vi "GEA2 Extract 2015 Washer.vi"(6 "ERD Cross Reference List":T1[][](array[typedef]) {"ERD Number" format="%.0x"}, 7 "Enable Diagnostic Data":T3, 8 "Error In":errorcluster, 9 "ERD Number":u16 format="%x", 10 "Data":string, 11 "ERD Headers":string[](array[string])) -> (0 "Error Out":errorcluster, 3 "Array":string[][](array[string]))   [LabVIEW 2016, in "GEA2_Toolkit.lvlib"]
uses:
  library/GEA2_Toolkit.lvlib
  Washer HCC/Washer HCC NEWFI/Type Definitions/HCC Washer Types.ctl
  type defs/ERD Read Data In.ctl
  type defs/Data Type.ctl
panel:
  in  "Header Array (Debug)":string[](array[string])=["Critical Major (0x0100)", "Critical Minor (0x0100)", "Non-Critical Major (0x0100)", "Non-Critical Minor (0x0100)", "Daily Revision (0x0100)", "Cycle Count (0x008E)", "XML Critical Major (0xF014)", "XML Critical Minor (0xF014)", "XML Non-Critical Major (0xF014)", "XML Non-Critical Minor (0xF014)", "Available Free Stack % (0xF026)", "Extra Rinse (0xF032)", "Deep Rinse_Fabric Softener (0xF033)", "My Cycle (0xF034)", "Soil Level (0x2015)", "Spin Level (0xF035)", "Stain (0xF036)", "Temperature Level (0xF037)", "Load Size (0xF038)", "Machine State (0xF039)", "Cycle Selected (0xF03B)", "Delay Time (0x2010)", "Soak Time (0xF03C)", "Auto Soak Level (0xF04B)", "Deep Fill (0xF04F)", "Warm Rinse (0xF050)", "Remaining Cycle Time(s) (0xF061)", "Wet Load Gallons (0xF068)", "Tub Volume Gallons (0xF069)", "Pressure (inches of H20) (0xF06A)", "Target Gallons (0xF06D)", "Load Type (0xF06E)", "Lid Switch (0xF06F)", "Hot Water Valve (0xF09C)", "Cold Water Valve (0xF09C)", "Spray_Rinse Valve (0xF09C)", "Fabric Softener Valve (0xF09C)", "Lid Lock Req State (0xF072)", "Lid Lock Status (0xF073)", "Cycle Engine State (0xF074)", "Current Water Temperature (°F) (0xF077)", "Drain Pump (0xF09A)", "Recirculating Pump (0xF079)", "Sub-Cycle (0xF07B)", "Target Level Inches (0xF07D)", "Valve Relay (0xF09B)", "Lid Lock FB (0xF080)", "Target Bath Temperature (°F) (0xF082)", "Current Bath Temperature (°F) (0xF083)", "Cold Inlet Temperature (°F) (0xF084)", "Hot Inlet Temperature (°F) (0xF085)", "Warm Inlet Temperature (°F) (0xF086)", "Hot Gallons (0xF087)", "Cold Gallons (0xF087)", "Hot Seg Valve Time (0xF088)", "Cold Seg Valve Time (0xF088)", "Child Safety (0xF089)", "Segment Gallons (0xF08A)", "Ramp Average Current (0xF09E)", "Coast Line Voltage (0xF09F)", "Ramp Speed (0xF0A0)", "Ramp Time (0xF0A1)", "Coast Time (0xF0A2)", "Dry Load Size (0xF0A3)", "Folding in Acceleration (0xF0A4)", "Max Jerk In Acceleration (0xF0A5)", "Max Jerk In S-S (0xF0A6)", "Shaft Speed (RPM) (0xF0A8)", "Basket Speed (RPM) (0xF0A9)", "Current RMS (Amps) (0xF0AB)", "Target Speed (RPM) (0xF0AC)", "Motor Mode (0xF0B1)", "OOB Detected in Acceleration (0xF0B3)", "OOB Detected in S-S (0xF0B4)", "OOB ReDistribution Required (0xF0B5)", "Motor Profile Status (0xF0B7)", "Motor Profile (0xF0B7)", "Mode Shift Status (0xFF22)", "ME Relay (0xF0BE)", "Mode Shift FB (0xF0BF)", "MS Motor (0xF0C0)", "Partial Coast Time (0xF0C6)", "Ramp Line Voltage (0xF0C7)", "Personality (0xFF00)", "Reset Source (0xFF02)", "DC Bus Voltage RMS value (0xF0C4)"]
  out "ERD Number 2":u16 format="%x"
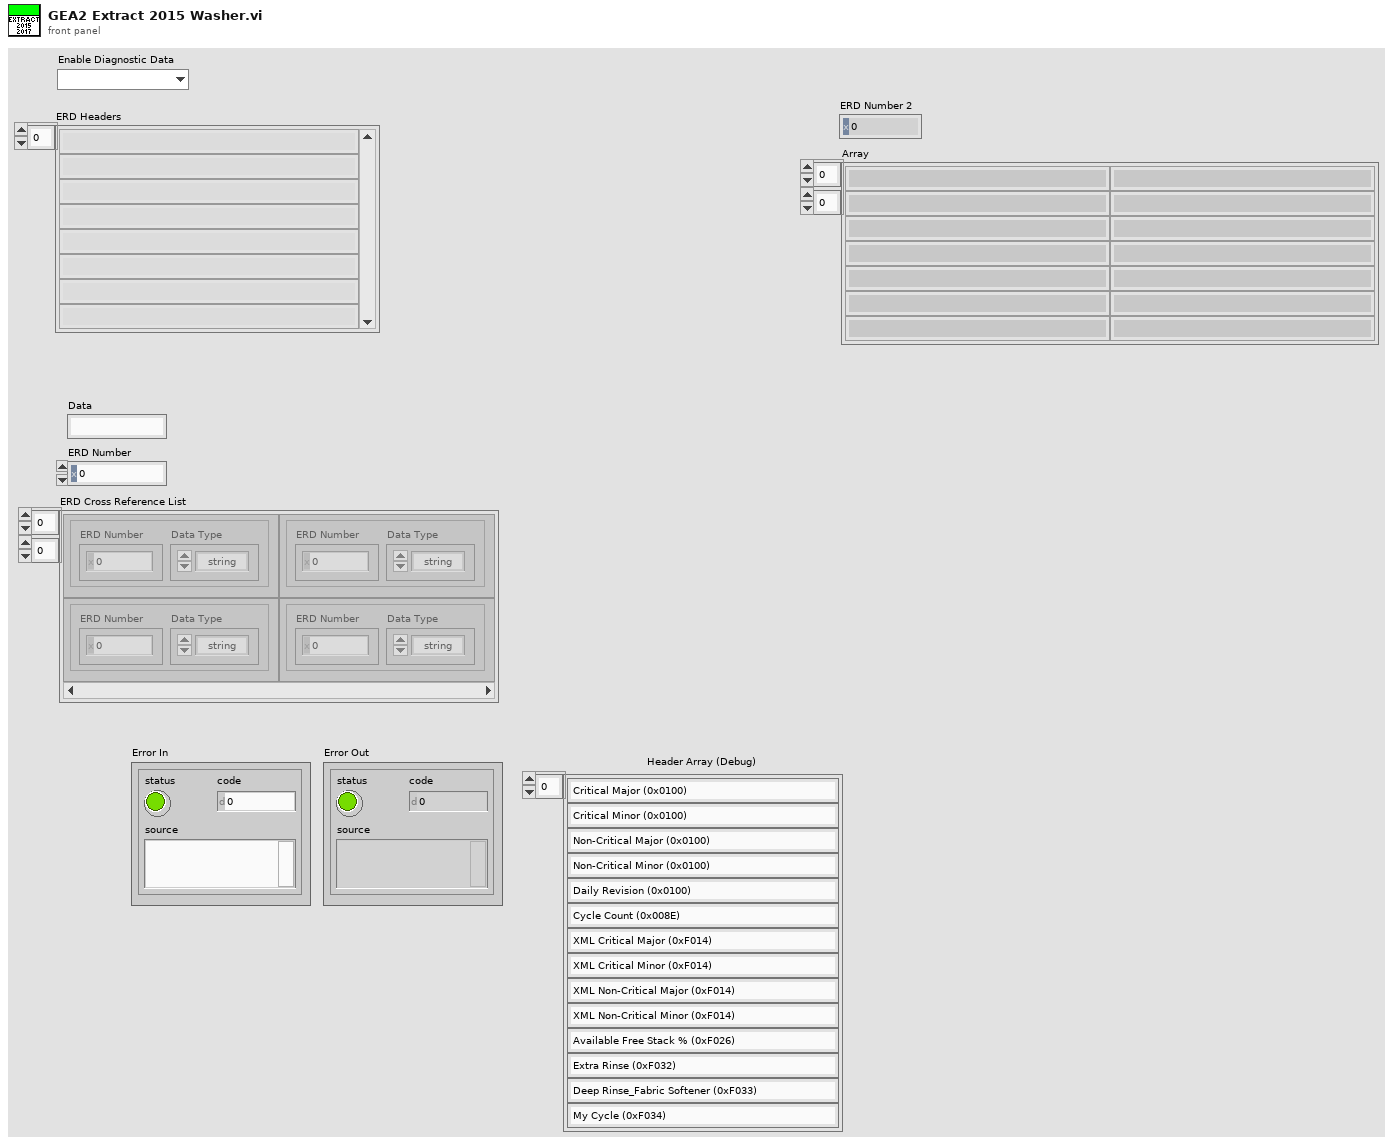
[diagram p1: front panel]
types:
  T1 = typedef "GEA2_Toolkit.lvlib/ERD Read Data In.ctl" = cluster{"ERD Number":u16, "Data Type":T2}
  T2 = typedef "GEA2_Toolkit.lvlib/Data Type.ctl" = enum16{"string", "boolean", "uint8_t", "uint16_t", "uint32_t", "uint64_t"}
  T3 = typedef "HCC Washer Types.ctl" = enum16{"", "Viper Washer", "Hawk Washer", "2015 Washer", "2017 Washer"}
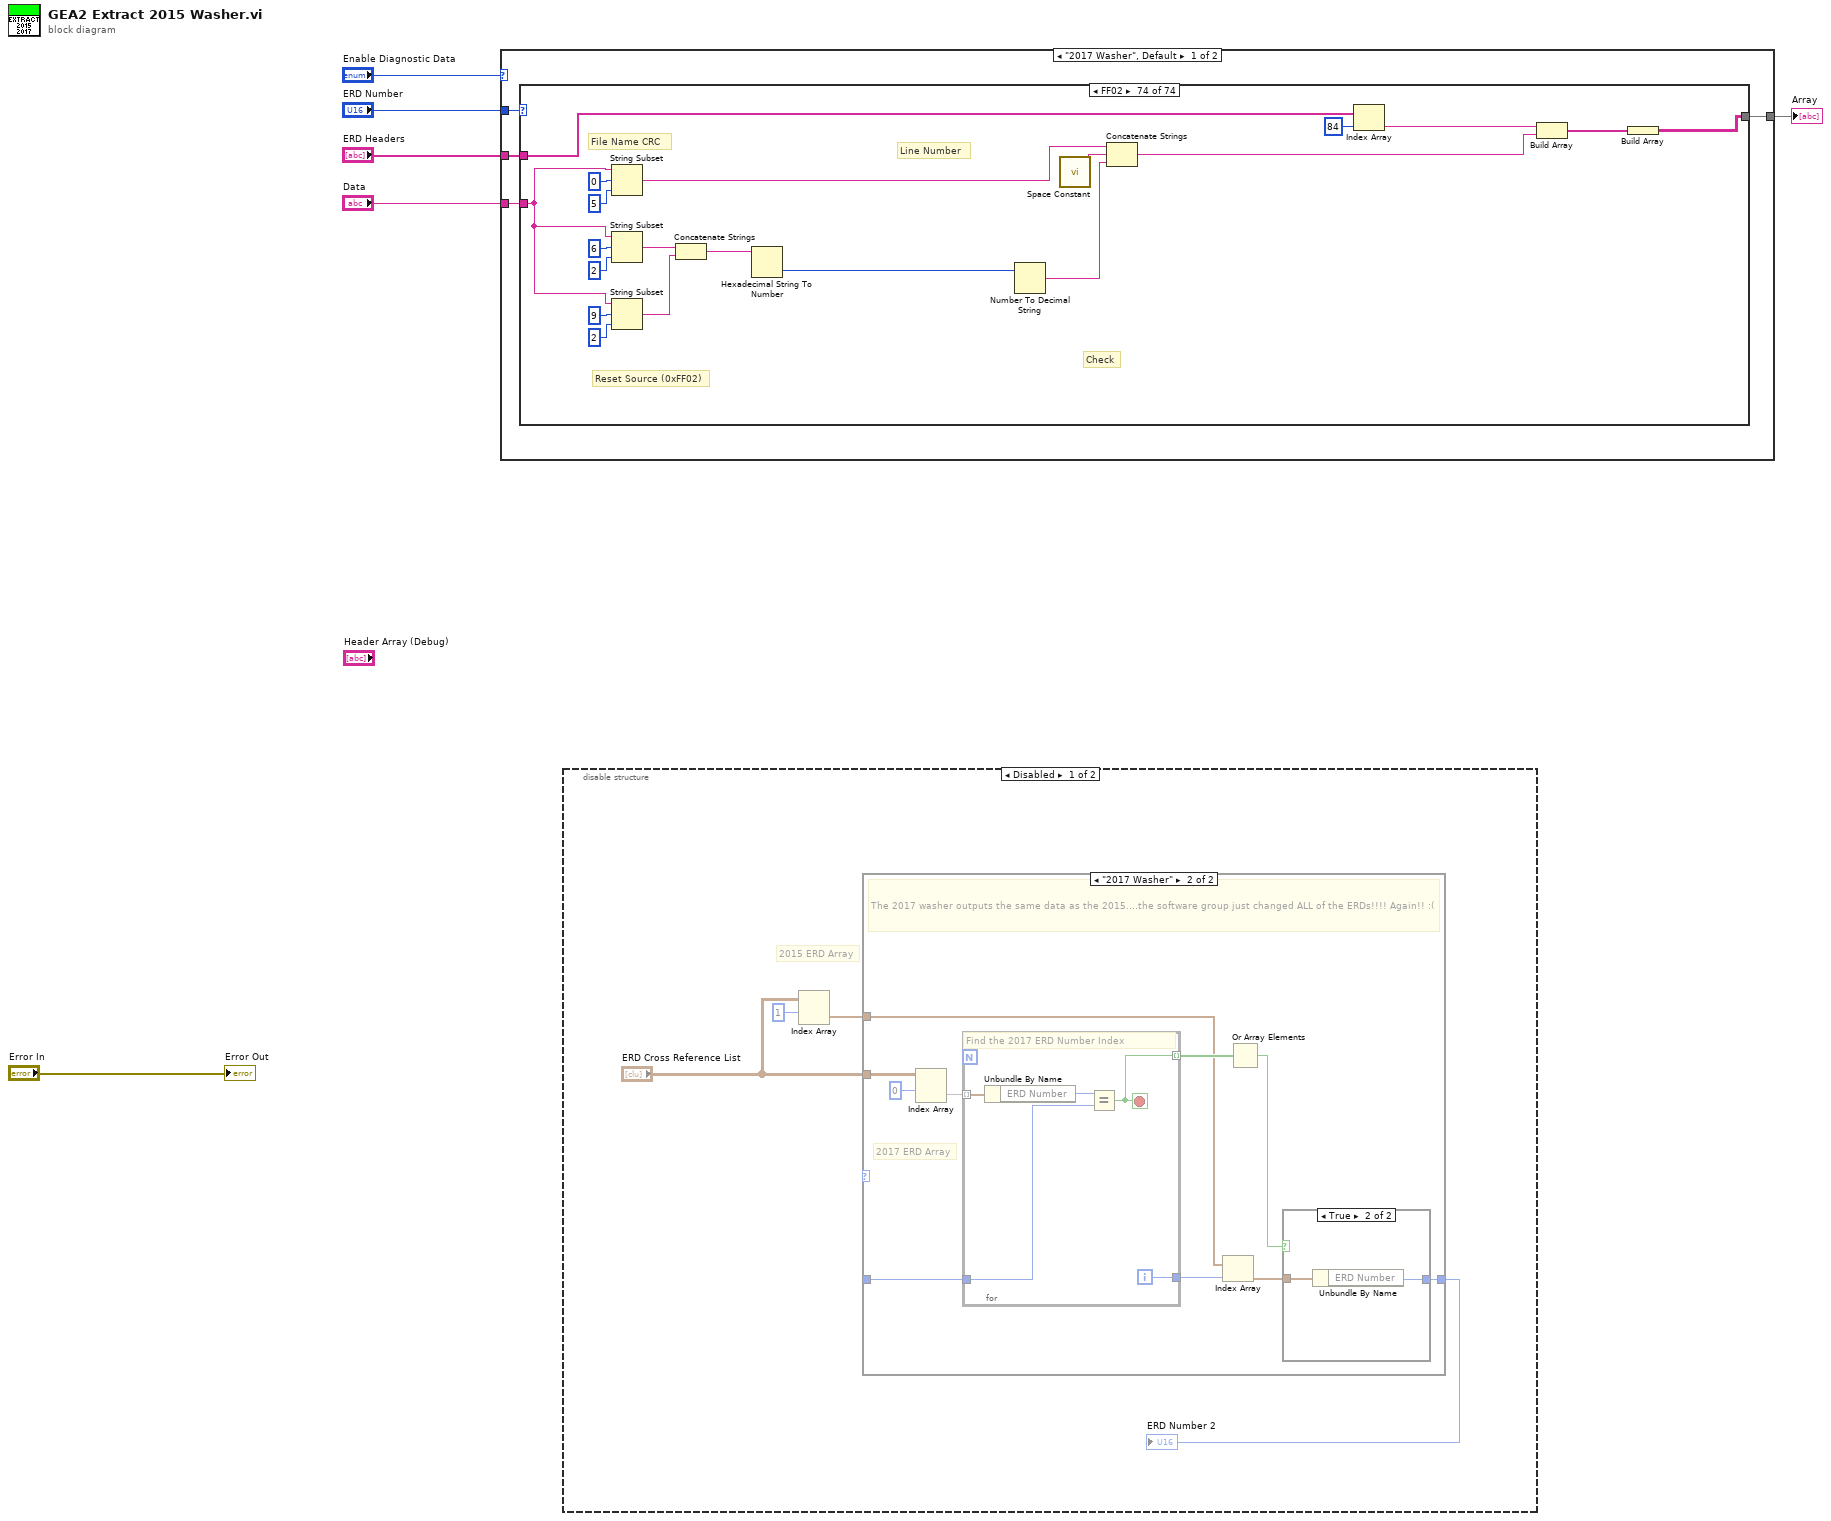
[diagram p0: block diagram]
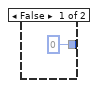
[diagram p3: hidden frame]
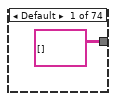
[diagram p5: hidden frame]
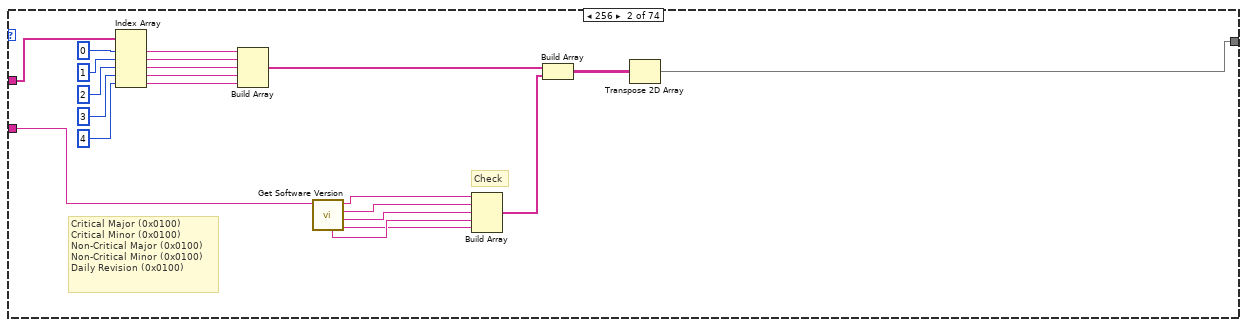
[diagram p6: hidden frame]
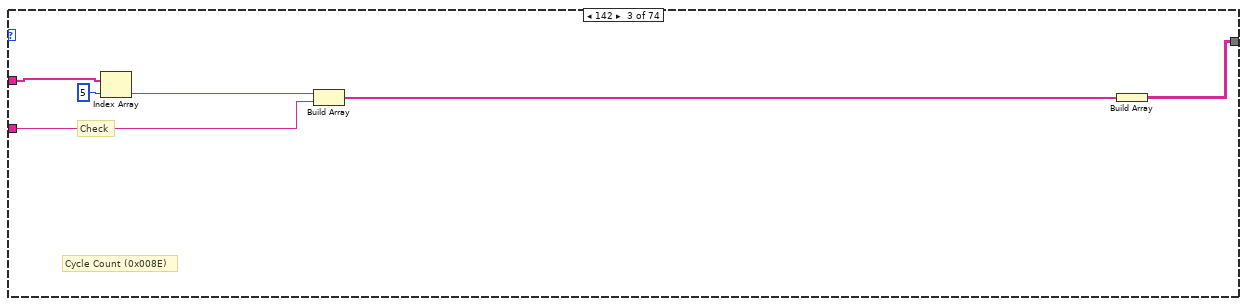
[diagram p7: hidden frame]
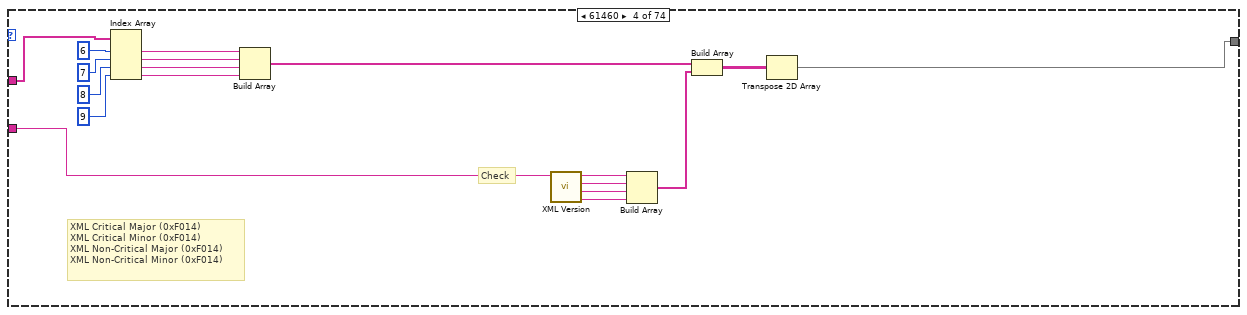
[diagram p8: hidden frame]
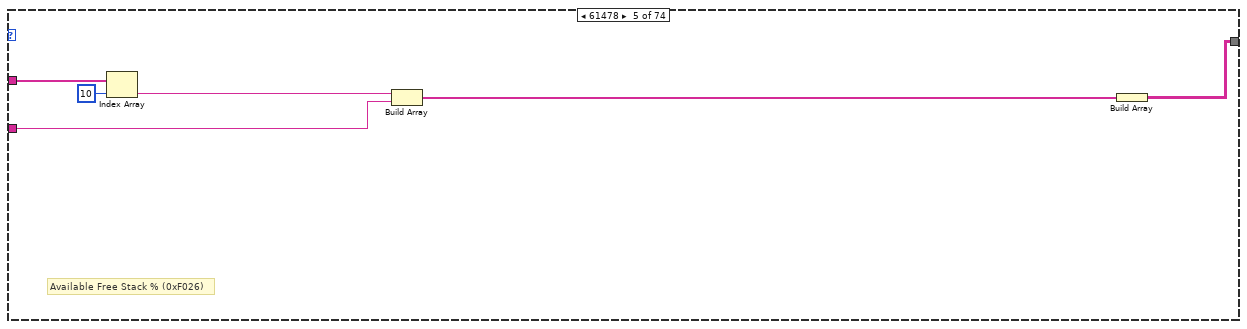
[diagram p9: hidden frame]
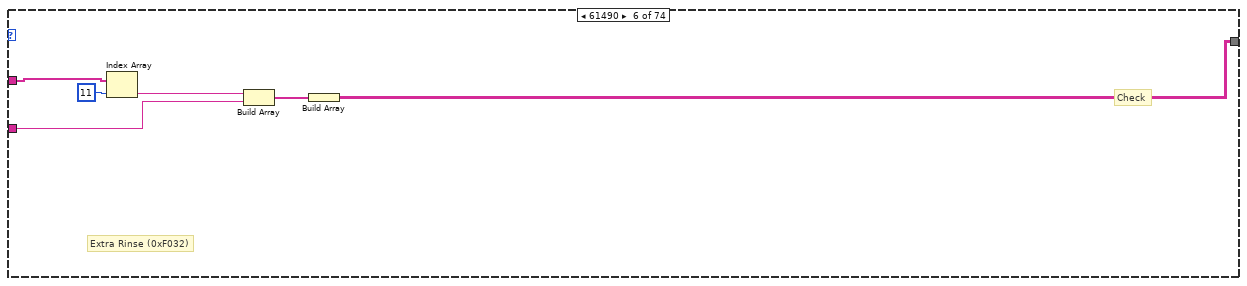
[diagram p10: hidden frame]
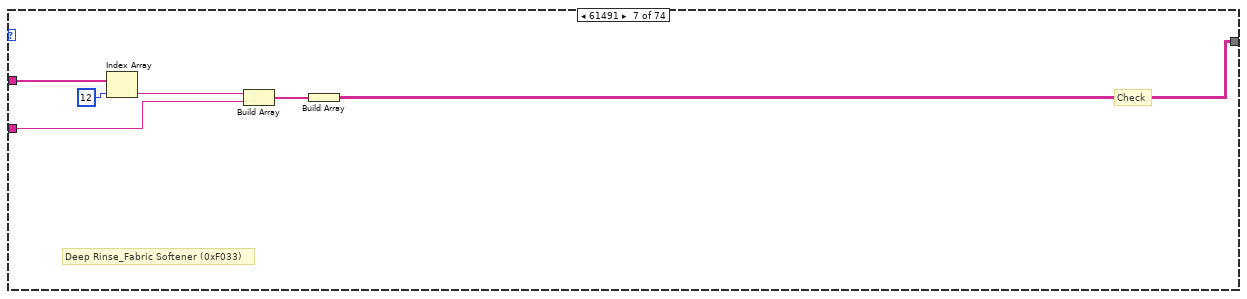
[diagram p11: hidden frame]
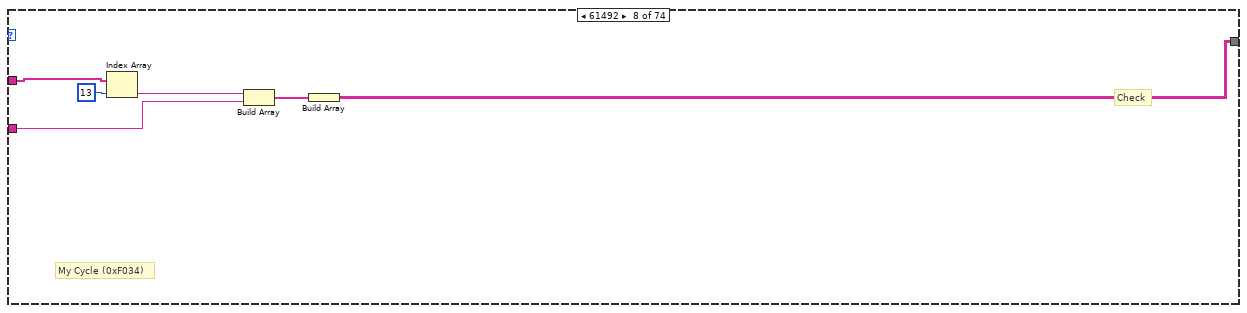
[diagram p12: hidden frame]
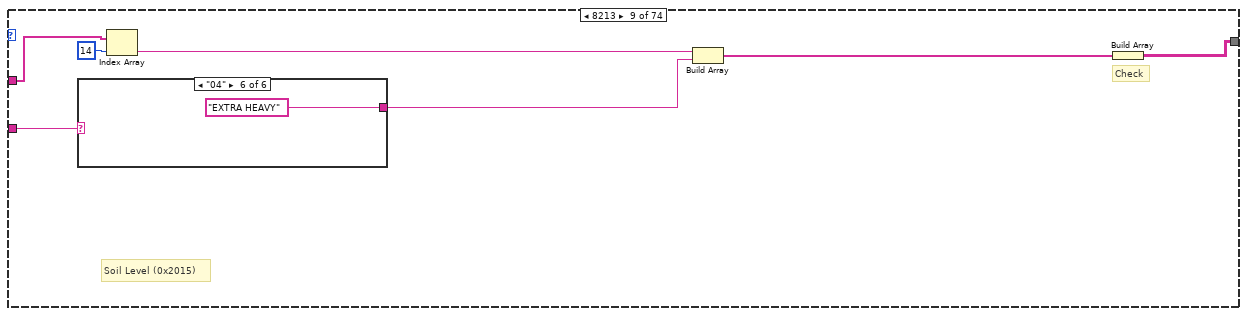
[diagram p13: hidden frame]
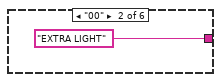
[diagram p15: hidden frame]
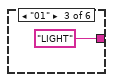
[diagram p16: hidden frame]
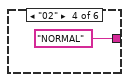
[diagram p17: hidden frame]
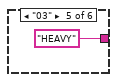
[diagram p18: hidden frame]
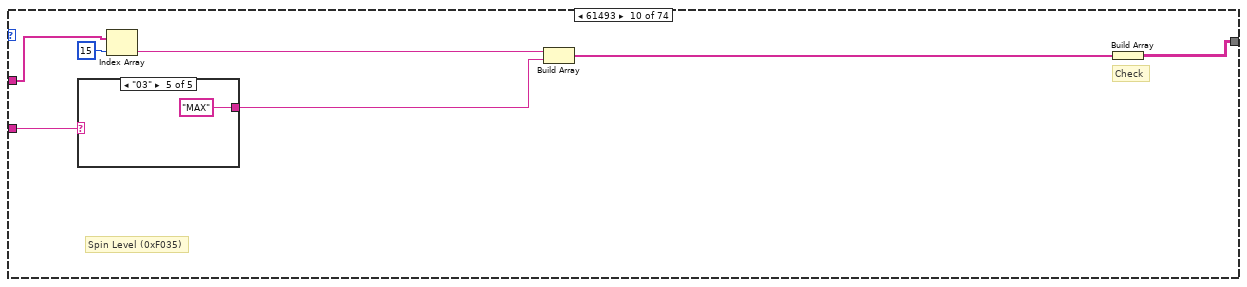
[diagram p19: hidden frame]
diagram:
  n1 = case shown="\"2017 Washer\", Default" "Enable Diagnostic Data" {
    tunnel: [w8 w808] -> w6
    tunnel: "ERD Headers" -> [w10 w807]
    tunnel: "Data" -> [w9 w806]
    tunnel: "ERD Number" -> [w7 w805]
    frame "2017 Washer", Default {
      n2 = case shown="FF02" w7 {
        tunnel: w9 -> [_ w32 w33 w56 w57 w63 w69 w75 w87 w100 w112 w126 w140 w153 w161 w179 w185 w192 w203 w210 w216 w223 w234 w245 w256 w272 w286 w317 w327 w340 w346 w353 w368 w378 w388 w397 w413 w423 w428 w438 w448 w458 w468 w490 w504 w505 w512 w522 w531 w538 w544 w550 w557 w570 w592 w614 w629 w635 w642 w658 w675 w684 w690 w696 w713 w734 w741 w747 w753 w765 w766 w773 w779 w795]
        tunnel: [string[][] [] w12 w34 w39 w58 w64 w70 w76 w81 w94 w106 w120 w134 w147 w155 w180 w186 w191 w197 w211 w217 w228 w235 w246 w257 w266 w288 w292 w320 w334 w347 w354 w362 w372 w382 w398 w407 w417 w429 w439 w449 w459 w469 w477 w491 w507 w515 w523 w532 w539 w545 w551 w558 w563 w585 w607 w630 w636 w643 w651 w669 w685 w691 w697 w702 w728 w742 w748 w754 w760 w767 w774 w780 w785] -> w8
        tunnel: w10 -> [_ w14 w38 w55 w62 w68 w71 w77 w83 w96 w107 w122 w136 w149 w157 w181 w187 w193 w199 w212 w218 w229 w236 w247 w259 w268 w289 w297 w323 w335 w348 w357 w363 w374 w384 w402 w408 w419 w432 w442 w450 w460 w472 w482 w496 w506 w516 w526 w534 w540 w546 w552 w559 w566 w586 w610 w631 w637 w644 w652 w671 w686 w692 w698 w705 w730 w743 w749 w755 w761 w768 w775 w781 w786]
        frame Default {
        }
        frame 256 {
          # "Critical Major (0x0100)\nCritical Minor (0x0100)\nNon-Critical Major (0x0100)\nNon-Critical Minor (0x0100)\nDaily Revision (0x0100)"
          # "Check"
          n3 = Index Array(array=w14, index #1=0 ("index"), index #2=1 ("index"), index #3=2 ("index"), index #4=3 ("index"), index #5=4 ("index")) -> (element #1=w26:string, element #2=w25:string, element #3=w24:string, element #4=w23:string, element #5=w22:string)
          n4 = Build Array(w26, w25, w24, w23, w22) -> (w16:string[])
          n5 = call "Get Software Version.vi"("Data"=w32) -> ("Daily Revision"=w17:string, "Non-Critical Major"=w19:string, "Critical Minor"=w20:string, "Critical Major"=w21:string, "Non-Critical Minor"=w18:string)  [unwired: 6 in]
          n6 = Build Array(w21, w20, w19, w18, w17) -> (w15:string[])
          n7 = Build Array(w16, w15) -> (w13:string[][])
          n8 = Transpose 2D Array(2D array=w13) -> (transposed array=w12:string[][])
        }
        frame 142 {
          # "Cycle Count (0x008E)"
          # "Check"
          n9 = Index Array(array=w38, index=5) -> (element=w36:string)
          n10 = Build Array(w36, w33) -> (w35:string[])
          n11 = Build Array(w35) -> (w34:string[][])
        }
        frame 61460 {
          # "XML Critical Major (0xF014)\nXML Critical Minor (0xF014)\nXML Non-Critical Major (0xF014)\nXML Non-Critical Minor (0xF014)"
          # "Check"
          n12 = Index Array(array=w55, index #1=6 ("index"), index #2=7 ("index"), index #3=8 ("index"), index #4=9 ("index")) -> (element #1=w50:string, element #2=w49:string, element #3=w48:string, element #4=w47:string)
          n13 = Build Array(w50, w49, w48, w47) -> (w42:string[])
          n14 = call "XML Version.vi"("Data"=w56) -> ("XML Non-Critical Minor"=w43:string, "XML Non-Critical Major"=w44:string, "XML Critical Minor"=w45:string, "XML Critical Major"=w46:string)  [unwired: 7 in]
          n15 = Build Array(w46, w45, w44, w43) -> (w41:string[])
          n16 = Build Array(w42, w41) -> (w40:string[][])
          n17 = Transpose 2D Array(2D array=w40) -> (transposed array=w39:string[][])
        }
        frame 61478 {
          # "Available Free Stack % (0xF026)"
          n18 = Index Array(array=w62, index=10) -> (element=w60:string)
          n19 = Build Array(w60, w57) -> (w59:string[])
          n20 = Build Array(w59) -> (w58:string[][])
        }
        frame 61490 {
          # "Extra Rinse (0xF032)"
          # "Check"
          n21 = Index Array(array=w68, index=11) -> (element=w66:string)
          n22 = Build Array(w66, w63) -> (w65:string[])
          n23 = Build Array(w65) -> (w64:string[][])
        }
        frame 61491 {
          # "Deep Rinse_Fabric Softener (0xF033)"
          # "Check"
          n24 = Index Array(array=w71, index=12) -> (element=w73:string)
          n25 = Build Array(w73, w69) -> (w72:string[])
          n26 = Build Array(w72) -> (w70:string[][])
        }
        frame 61492 {
          # "My Cycle (0xF034)"
          # "Check"
          n27 = Index Array(array=w77, index=13) -> (element=w79:string)
          n28 = Build Array(w79, w75) -> (w78:string[])
          n29 = Build Array(w78) -> (w76:string[][])
        }
        frame 8213 {
          # "Soil Level (0x2015)"
          # "Check"
          n30 = case shown="\"04\"" w87 {
            selector: w87 -> [w88 _ _ _ _ _]
            tunnel: [w88 "EXTRA LIGHT" "LIGHT" "NORMAL" "HEAVY" "EXTRA HEAVY"] -> w82
            frame Default {
            }
            frame "00" {
            }
            frame "01" {
            }
            frame "02" {
            }
            frame "03" {
            }
            frame "04" {
            }
          }
          n31 = Index Array(array=w83, index=14) -> (element=w85:string)
          n32 = Build Array(w85, w82) -> (w84:string[])
          n33 = Build Array(w84) -> (w81:string[][])
        }
        frame 61493 {
          # "Spin Level (0xF035)"
          # "Check"
          n34 = case shown="\"03\"" w100 {
            selector: w100 -> [w101 _ _ _ _]
            tunnel: [w101 "NO SPIN" "NORMAL" "MORE " "MAX"] -> w95
            frame Default {
            }
            frame "00" {
            }
            frame "01" {
            }
            frame "02" {
            }
            frame "03" {
            }
          }
          n35 = Index Array(array=w96, index=15) -> (element=w98:string)
          n36 = Build Array(w98, w95) -> (w97:string[])
          n37 = Build Array(w97) -> (w94:string[][])
        }
        frame 61494 {
          # "Stain (0xF036)"
          # "Check"
          n38 = case shown="\"01\"" w112 {
            selector: w112 -> [w113 _ _ _ _ _ _]
            tunnel: [w113 "OFF" "TOMATO" "WINE" "BLOOD" "GRASS" "DIRT"] -> w108
            frame Default {
            }
            frame "00" {
            }
            frame "01" {
            }
            frame "02" {
            }
            frame "03" {
            }
            frame "04" {
            }
            frame "05" {
            }
          }
          n39 = Index Array(array=w107, index=16) -> (element=w110:string)
          n40 = Build Array(w110, w108) -> (w109:string[])
          n41 = Build Array(w109) -> (w106:string[][])
        }
        frame 61495 {
          # "Temperature Level (0xF037)"
          n42 = case shown="\"05\"" w126 {
            selector: w126 -> [w127 _ _ _ _ _ _]
            tunnel: [w127 "TAP COLD" "COLD" "COOL" "COLORS" "WARM" "HOT"] -> w121
            frame Default {
            }
            frame "00" {
            }
            frame "01" {
            }
            frame "02" {
            }
            frame "03" {
            }
            frame "04" {
            }
            frame "05" {
            }
          }
          n43 = Index Array(array=w122, index=17) -> (element=w124:string)
          n44 = Build Array(w124, w121) -> (w123:string[])
          n45 = Build Array(w123) -> (w120:string[][])
        }
        frame 61496 {
          # "Load Size (0xF038)"
          # "Check"
          n46 = case shown="\"04\"" w140 {
            selector: w140 -> [w141 _ _ _ _ _]
            tunnel: [w141 "SMALL" "MEDIUM" "LARGE" "SUPER" "PRECISE FILL"] -> w135
            frame Default {
            }
            frame "00" {
            }
            frame "01" {
            }
            frame "02" {
            }
            frame "03" {
            }
            frame "04" {
            }
          }
          n47 = Index Array(array=w136, index=18) -> (element=w138:string)
          n48 = Build Array(w138, w135) -> (w137:string[])
          n49 = Build Array(w137) -> (w134:string[][])
        }
        frame 61497 {
          # "Machine State (0xF039)"
          # "Check"
          n50 = Decimal String To Number(string=w153) -> (number=w154:i32)  [unwired: 2 in, 1 out]
          n51 = Index Array(array=w149, index=19) -> (element=w151:string)
          n52 = call "Machine State.vi"("Numeric"=w154) -> ("Profile Status"=w148:string)  [unwired: 10 in]
          n53 = Build Array(w151, w148) -> (w150:string[])
          n54 = Build Array(w150) -> (w147:string[][])
        }
        frame 61499 {
          # "Cycle Selected (0xF03B)"
          # "Check"
          n55 = Decimal String To Number(string=w161) -> (number=w162:i32)  [unwired: 2 in, 1 out]
          n56 = Index Array(array=w157, index=20) -> (element=w159:string)
          n57 = case shown="6" w162 {
            tunnel: ["Cycle 0" ("Motor Profile") "Cycle 1" ("Motor Profile") "Cycle 2" ("Motor Profile") "Cycle 3" ("Motor Profile") "Cycle 4" ("Motor Profile") "Cycle 5" ("Motor Profile") "Cycle 6" ("Motor Profile") "Cycle 7" ("Motor Profile") "Cycle 8" ("Motor Profile") "Cycle 9" ("Motor Profile") "Cycle 10" ("Motor Profile") "Cycle 11" ("Motor Profile") "Cycle 12" ("Motor Profile") "Cycle 13" ("Motor Profile") "Cycle 14" ("Motor Profile") "Cycle 15" ("Motor Profile")] -> w156
            frame 0, Default {
            }
            frame 1 {
            }
            frame 2 {
            }
            frame 3 {
            }
            frame 4 {
            }
            frame 5 {
            }
            frame 6 {
            }
            frame 7 {
            }
            frame 8 {
            }
            frame 9 {
            }
            frame 10 {
            }
            frame 11 {
            }
            frame 12 {
            }
            frame 13 {
            }
            frame 14 {
            }
            frame 15 {
            }
          }
          n58 = Build Array(w159, w156) -> (w158:string[])
          n59 = Build Array(w158) -> (w155:string[][])
        }
        frame 8208 {
          # "Delay Time (0x2010)"
          # "Might not work"
          n60 = Index Array(array=w181, index=21) -> (element=w183:string)
          n61 = Build Array(w183, w179) -> (w182:string[])
          n62 = Build Array(w182) -> (w180:string[][])
        }
        frame 61500 {
          # "Soak Time (0xF03C)"
          # "Check"
          n63 = Index Array(array=w187, index=22) -> (element=w189:string)
          n64 = Build Array(w189, w185) -> (w188:string[])
          n65 = Build Array(w188) -> (w186:string[][])
        }
        frame 61515 {
          # "Auto Soak Level (0xF04B)"
          # "Check"
          n66 = Index Array(array=w193, index=23) -> (element=w195:string)
          n67 = Build Array(w195, w192) -> (w194:string[])
          n68 = Build Array(w194) -> (w191:string[][])
        }
        frame 61519 {
          # "Deep Fill (0xF04F)"
          # "Check. Could add names:\n00=Off\n01=Incremental Fill\n02=Max Fill"
          n69 = case shown="\"00\", Default" w203 {
            tunnel: [FALSE ("Eco Wash") TRUE ("Eco Wash") TRUE ("Eco Wash")] -> _
            tunnel: ["Off" "Incremental Fill" "Max Fill"] -> w198
            frame "00", Default {
            }
            frame "01" {
            }
            frame "02" {
            }
          }
          n70 = Index Array(array=w199, index=24) -> (element=w201:string)
          n71 = Build Array(w201, w198) -> (w200:string[])
          n72 = Build Array(w200) -> (w197:string[][])
        }
        frame 61520 {
          # "Warm Rinse (0xF050)"
          # "Check"
          n73 = Index Array(array=w212, index=25) -> (element=w214:string)
          n74 = Build Array(w214, w210) -> (w213:string[])
          n75 = Build Array(w213) -> (w211:string[][])
        }
        frame 61537 {
          # "Remaining Cycle Time(s) (0xF061)"
          # "Check"
          n76 = Index Array(array=w218, index=26) -> (element=w220:string)
          n77 = Build Array(w220, w216) -> (w219:string[])
          n78 = Build Array(w219) -> (w217:string[][])
        }
        frame 61544 {
          # "Wet Load Gallons (0xF068)"
          # "Check"
          n79 = Fract/Exp String To Number(string=w223) -> (number=w222:dbl)  [unwired: 3 in, 1 out]
          n80 = Index Array(array=w229, index=27) -> (element=w231:string)
          n81 = Divide(x=w222, y=100.0) -> (x/y=w227:dbl)
          n82 = Number To Fractional String(number=w227, precision (6)=i16 3) -> (F-format string=w224:string)  [unwired: 2 in]
          n83 = Build Array(w231, w224) -> (w230:string[])
          n84 = Build Array(w230) -> (w228:string[][])
        }
        frame 61545 {
          # "Tub Volume Gallons (0xF069)"
          # "Check"
          n85 = Fract/Exp String To Number(string=w234) -> (number=w233:dbl)  [unwired: 3 in, 1 out]
          n86 = Index Array(array=w236, index=28) -> (element=w241:string)
          n87 = Divide(x=w233, y=100.0) -> (x/y=w237:dbl)
          n88 = Number To Fractional String(number=w237, precision (6)=i16 3) -> (F-format string=w238:string)  [unwired: 2 in]
          n89 = Build Array(w241, w238) -> (w240:string[])
          n90 = Build Array(w240) -> (w235:string[][])
        }
        frame 61546 {
          # "Pressure (inches of H20) (0xF06A)"
          n91 = Fract/Exp String To Number(string=w245) -> (number=w244:dbl)  [unwired: 3 in, 1 out]
          n92 = Index Array(array=w247, index=29) -> (element=w252:string)
          n93 = Divide(x=w244, y=1000.0) -> (x/y=w248:dbl)
          n94 = Number To Fractional String(number=w248, precision (6)=i16 3) -> (F-format string=w249:string)  [unwired: 2 in]
          n95 = Build Array(w252, w249) -> (w251:string[])
          n96 = Build Array(w251) -> (w246:string[][])
        }
        frame 61549 {
          # "Target Gallons (0xF06D)"
          # "Check"
          n97 = Fract/Exp String To Number(string=w256) -> (number=w255:dbl)  [unwired: 3 in, 1 out]
          n98 = Index Array(array=w259, index=30) -> (element=w263:string)
          n99 = Divide(x=w255, y=100.0) -> (x/y=w258:dbl)
          n100 = Number To Fractional String(number=w258, precision (6)=i16 3) -> (F-format string=w260:string)  [unwired: 2 in]
          n101 = Build Array(w263, w260) -> (w262:string[])
          n102 = Build Array(w262) -> (w257:string[][])
        }
        frame 61550 {
          # "Load Type (0xF06E)"
          # "Check....could use the U8 conversion"
          n103 = case shown="\"3\"" w272 {
            selector: w272 -> [w273 _ _ _ _ _ _ _ _ _ _ _ _]
            tunnel: [w273 "UNKNOWN" "COTTON" "SYNTHETIC" "MIXED" "WET" "LOW FLOW" "SMALL" "MEDIUM" "LARGE" "SUPER" "SUPER PLUS" "MAX"] -> w267
            frame Default {
            }
            frame "0" {
            }
            frame "1" {
            }
            frame "2" {
            }
            frame "3" {
            }
            frame "4" {
            }
            frame "5" {
            }
            frame "6" {
            }
            frame "7" {
            }
            frame "8" {
            }
            frame "9" {
            }
            frame "10" {
            }
            frame "11" {
            }
          }
          n104 = Index Array(array=w268, index=31) -> (element=w270:string)
          n105 = Build Array(w270, w267) -> (w269:string[])
          n106 = Build Array(w269) -> (w266:string[][])
        }
        frame 61551 {
          # "Lid Switch (0xF06F)"
          # "Check"
          n107 = Index Array(array=w289, index=32) -> (element=w291:string)
          n108 = Build Array(w291, w286) -> (w290:string[])
          n109 = Build Array(w290) -> (w288:string[][])
        }
        frame 61596 {
          # "Hot Water Valve (0xF09C)\nCold Water Valve (0xF09C)\nSpray_Rinse Valve (0xF09C)\nFabric Softener Valve (0xF09C)"
          # "Check"
          n110 = Index Array(array=w297, index #1=33 ("index"), index #2=34 ("index"), index #3=35 ("index"), index #4=36 ("index")) -> (element #1=w304:string, element #2=w303:string, element #3=w302:string, element #4=w301:string)
          n111 = Build Array(w304, w303, w302, w301) -> (w300:string[])
          n112 = Decimal String To Number(string=w317) -> (number=w318:i32)  [unwired: 2 in, 1 out]
          n113 = Number To Boolean Array(number=w318) -> (Boolean array=w319:bool[])
          n114 = Index Array(array=w319) -> (element #1=w312:bool, element #2=w311:bool, element #3=w310:bool, element #4=w309:bool)  [unwired: 4 in]
          n115 = Boolean To (0,1)(Boolean=w312) -> (0, 1=w316:i16)
          n116 = Boolean To (0,1)(Boolean=w311) -> (0, 1=w315:i16)
          n117 = Boolean To (0,1)(Boolean=w310) -> (0, 1=w314:i16)
          n118 = Boolean To (0,1)(Boolean=w309) -> (0, 1=w313:i16)
          n119 = Number To Decimal String(number=w316) -> (decimal integer string=w296:string)  [unwired: 1 in]
          n120 = Number To Decimal String(number=w315) -> (decimal integer string=w295:string)  [unwired: 1 in]
          n121 = Number To Decimal String(number=w314) -> (decimal integer string=w294:string)  [unwired: 1 in]
          n122 = Number To Decimal String(number=w313) -> (decimal integer string=w293:string)  [unwired: 1 in]
          n123 = Build Array(w296, w295, w294, w293) -> (w299:string[])
          n124 = Build Array(w300, w299) -> (w298:string[][])
          n125 = Transpose 2D Array(2D array=w298) -> (transposed array=w292:string[][])
        }
        frame 61554 {
          # "Lid Lock Req State (0xF072)"
          # "Check"
          n126 = String Subset(string=w327, offset (0)=3, length (rest)=2 ("length (rest)")) -> (substring=w328:string)
          n127 = Index Array(array=w323, index=37) -> (element=w325:string)
          n128 = Hexadecimal String To Number(string=w328) -> (number=w326:u32)  [unwired: 2 in, 1 out]
          n129 = case shown="0, Default" w326 {
            tunnel: ["UNLOCKED" "LOCKED" "FAILURE"] -> w321
            frame 0, Default {
            }
            frame 1 {
            }
            frame 2 {
            }
          }
          n130 = Build Array(w325, w321) -> (w324:string[])
          n131 = Build Array(w324) -> (w320:string[][])
        }
        frame 61555 {
          # "Lid Lock Status (0xF073)"
          # "Check"
          n132 = Decimal String To Number(string=w340) -> (number=w341:i32)  [unwired: 2 in, 1 out]
          n133 = Index Array(array=w335, index=38) -> (element=w338:string)
          n134 = case shown="2" w341 {
            tunnel: ["Unlocked" ("Motor Profile") "Locked" ("Motor Profile") "Failure" ("Motor Profile")] -> w336
            frame 0, Default {
            }
            frame 1 {
            }
            frame 2 {
            }
          }
          n135 = Build Array(w338, w336) -> (w337:string[])
          n136 = Build Array(w337) -> (w334:string[][])
        }
        frame 61556 {
          # "Cycle Engine State (0xF074)"
          n137 = call "Cycle Engine State.vi"("Data"=w346) -> ("Cycle Engine State"=w345:string)  [unwired: 10 in]
          n138 = Index Array(array=w348, index=39) -> (element=w350:string)
          n139 = Build Array(w350, w345) -> (w349:string[])
          n140 = Build Array(w349) -> (w347:string[][])
        }
        frame 61559 {
          # "Current Water Temperature (°F) (0xF077)"
          # "Check"
          n141 = Fract/Exp String To Number(string=w353) -> (number=w352:dbl)  [unwired: 3 in, 1 out]
          n142 = Index Array(array=w357, index=40) -> (element=w359:string)
          n143 = Divide(x=w352, y=10.0) -> (x/y=w356:dbl)
          n144 = Number To Fractional String(number=w356) -> (F-format string=w355:string)  [unwired: 3 in]
          n145 = Build Array(w359, w355) -> (w358:string[])
          n146 = Build Array(w358) -> (w354:string[][])
        }
        frame 61594 {
          # "Drain Pump (0xF09A)"
          # "Check"
          n147 = String Subset(string=w368, offset (0)=3, length (rest)=2 ("length (rest)")) -> (substring=w369:string)
          n148 = Index Array(array=w363, index=41) -> (element=w366:string)
          n149 = call "HexStringToBoolean.vi"("Hex String"=w369) -> ("decimal integer string"=w364:string)  [unwired: 1 in, 1 out]
          n150 = Build Array(w366, w364) -> (w365:string[])
          n151 = Build Array(w365) -> (w362:string[][])
        }
        frame 61561 {
          # "Recirculating Pump (0xF079)"
          n152 = String Subset(string=w378, offset (0)=3, length (rest)=2 ("length (rest)")) -> (substring=w379:string)
          n153 = Index Array(array=w374, index=42) -> (element=w376:string)
          n154 = call "HexStringToBoolean.vi"("Hex String"=w379) -> ("decimal integer string"=w373:string)  [unwired: 1 in, 1 out]
          n155 = Build Array(w376, w373) -> (w375:string[])
          n156 = Build Array(w375) -> (w372:string[][])
        }
        frame 61563 {
          # "Sub-Cycle (0xF07B)"
          # "Check"
          n157 = case shown="\"04\"" w388 {
            selector: w388 -> [w389 _ _ _ _ _ _]
            tunnel: [w389 "NONE" "FILL" "SOAK" "WASH" "RINSE" "SPIN"] -> w383
            frame Default {
            }
            frame "00" {
            }
            frame "01" {
            }
            frame "02" {
            }
            frame "04" {
            }
            frame "08" {
            }
            frame "10" {
            }
          }
          n158 = Index Array(array=w384, index=43) -> (element=w386:string)
          n159 = Build Array(w386, w383) -> (w385:string[])
          n160 = Build Array(w385) -> (w382:string[][])
        }
        frame 61565 {
          # "Target Level Inches (0xF07D)"
          # "Check"
          n161 = Fract/Exp String To Number(string=w397) -> (number=w396:dbl)  [unwired: 3 in, 1 out]
          n162 = Index Array(array=w402, index=44) -> (element=w404:string)
          n163 = Divide(x=w396, y=1000.0) -> (x/y=w401:dbl)
          n164 = Number To Fractional String(number=w401, precision (6)=i16 3) -> (F-format string=w399:string)  [unwired: 2 in]
          n165 = Build Array(w404, w399) -> (w403:string[])
          n166 = Build Array(w403) -> (w398:string[][])
        }
        frame 61595 {
          # "Valve Relay (0xF09B)"
          # "Check"
          n167 = String Subset(string=w413, offset (0)=3, length (rest)=2 ("length (rest)")) -> (substring=w414:string)
          n168 = Index Array(array=w408, index=45) -> (element=w411:string)
          n169 = call "HexStringToBoolean.vi"("Hex String"=w414) -> ("decimal integer string"=w409:string)  [unwired: 1 in, 1 out]
          n170 = Build Array(w411, w409) -> (w410:string[])
          n171 = Build Array(w410) -> (w407:string[][])
        }
        frame 61568 {
          # "Lid Lock FB (0xF080)"
          # "Check"
          n172 = case shown="\"01\"" w423 {
            selector: w423 -> [w424 _ _]
            tunnel: [w424 "LOCKED" ("Motor Profile") "UNLOCKED" ("Motor Profile")] -> w418
            frame "0", Default {
            }
            frame "00" {
            }
            frame "01" {
            }
          }
          n173 = Index Array(array=w419, index=46) -> (element=w421:string)
          n174 = Build Array(w421, w418) -> (w420:string[])
          n175 = Build Array(w420) -> (w417:string[][])
        }
        frame 61570 {
          # "Target Bath Temperature (°F) (0xF082)"
          # "Check"
          n176 = Fract/Exp String To Number(string=w428) -> (number=w427:dbl)  [unwired: 3 in, 1 out]
          n177 = Index Array(array=w432, index=47) -> (element=w434:string)
          n178 = Divide(x=w427, y=10.0) -> (x/y=w431:dbl)
          n179 = Number To Fractional String(number=w431) -> (F-format string=w430:string)  [unwired: 3 in]
          n180 = Build Array(w434, w430) -> (w433:string[])
          n181 = Build Array(w433) -> (w429:string[][])
        }
        frame 61571 {
          # "Current Bath Temperature (°F) (0xF083)"
          # "Check"
          n182 = Fract/Exp String To Number(string=w438) -> (number=w437:dbl)  [unwired: 3 in, 1 out]
          n183 = Index Array(array=w442, index=48) -> (element=w444:string)
          n184 = Divide(x=w437, y=10.0) -> (x/y=w441:dbl)
          n185 = Number To Fractional String(number=w441) -> (F-format string=w440:string)  [unwired: 3 in]
          n186 = Build Array(w444, w440) -> (w443:string[])
          n187 = Build Array(w443) -> (w439:string[][])
        }
        frame 61572 {
          # "Cold Inlet Temperature (°F) (0xF084)"
          # "Check"
          n188 = Fract/Exp String To Number(string=w448) -> (number=w447:dbl)  [unwired: 3 in, 1 out]
          n189 = Index Array(array=w450, index=49) -> (element=w454:string)
          n190 = Divide(x=w447, y=10.0) -> (x/y=w452:dbl)
          n191 = Number To Fractional String(number=w452) -> (F-format string=w451:string)  [unwired: 3 in]
          n192 = Build Array(w454, w451) -> (w453:string[])
          n193 = Build Array(w453) -> (w449:string[][])
        }
        frame 61573 {
          # "Hot Inlet Temperature (°F) (0xF085)"
          # "Check"
          n194 = Fract/Exp String To Number(string=w458) -> (number=w457:dbl)  [unwired: 3 in, 1 out]
          n195 = Index Array(array=w460, index=50) -> (element=w464:string)
          n196 = Divide(x=w457, y=10.0) -> (x/y=w462:dbl)
          n197 = Number To Fractional String(number=w462) -> (F-format string=w461:string)  [unwired: 3 in]
          n198 = Build Array(w464, w461) -> (w463:string[])
          n199 = Build Array(w463) -> (w459:string[][])
        }
        frame 61574 {
          # "Warm Inlet Temperature (°F) (0xF086)"
          # "Check"
          n200 = Fract/Exp String To Number(string=w468) -> (number=w467:dbl)  [unwired: 3 in, 1 out]
          n201 = Index Array(array=w472, index=51) -> (element=w474:string)
          n202 = Divide(x=w467, y=10.0) -> (x/y=w471:dbl)
          n203 = Number To Fractional String(number=w471) -> (F-format string=w470:string)  [unwired: 3 in]
          n204 = Build Array(w474, w470) -> (w473:string[])
          n205 = Build Array(w473) -> (w469:string[][])
        }
        frame 61575 {
          # "Hot Gallons (0xF087)\nCold Gallons (0xF087)"
          # "Check"
          # "Check"
          n206 = call "Hot and Cold Gallons.vi"("Data"=w490) -> ("ColdGallons"=w480:dbl, "Hot Gallons"=w481:dbl)  [unwired: 9 in]
          n207 = Index Array(array=w482, index #1=52 ("index"), index #2=53 ("index")) -> (element #1=w487:string, element #2=w486:string)
          n208 = Number To Fractional String(number=w481) -> (F-format string=w479:string)  [unwired: 3 in]
          n209 = Number To Fractional String(number=w480) -> (F-format string=w478:string)  [unwired: 3 in]
          n210 = Build Array(w487, w486) -> (w485:string[])
          n211 = Build Array(w479, w478) -> (w484:string[])
          n212 = Build Array(w485, w484) -> (w483:string[][])
          n213 = Transpose 2D Array(2D array=w483) -> (transposed array=w477:string[][])
        }
        frame 61576 {
          # "Hot Seg Valve Time (0xF088)\nCold Seg Valve Time (0xF088)"
          # "Check"
          # "Check"
          n214 = Index Array(array=w496, index #1=54 ("index"), index #2=55 ("index")) -> (element #1=w501:string, element #2=w500:string)
          n215 = Build Array(w501, w500) -> (w499:string[])
          n216 = call "Segment Valve Time.vi"("Data"=w504) -> ("Cold Segment Valve Time"=w492:u16, "Hot Segment Valve Time"=w493:u16)  [unwired: 9 in]
          n217 = Number To Decimal String(number=w493) -> (decimal integer string=w495:string)  [unwired: 1 in]
          n218 = Number To Decimal String(number=w492) -> (decimal integer string=w494:string)  [unwired: 1 in]
          n219 = Build Array(w495, w494) -> (w498:string[])
          n220 = Build Array(w499, w498) -> (w497:string[][])
          n221 = Transpose 2D Array(2D array=w497) -> (transposed array=w491:string[][])
        }
        frame 61577 {
          # "Child Safety (0xF089)"
          # "Check"
          n222 = Index Array(array=w506, index=56) -> (element=w509:string)
          n223 = Build Array(w509, w505) -> (w508:string[])
          n224 = Build Array(w508) -> (w507:string[][])
        }
        frame 61578 {
          # "Segment Gallons (0xF08A)"
          # "Check"
          n225 = Fract/Exp String To Number(string=w512) -> (number=w511:dbl)  [unwired: 3 in, 1 out]
          n226 = Index Array(array=w516, index=57) -> (element=w518:string)
          n227 = Divide(x=w511, y=100.0) -> (x/y=w514:dbl)
          n228 = Number To Fractional String(number=w514) -> (F-format string=w513:string)  [unwired: 3 in]
          n229 = Build Array(w518, w513) -> (w517:string[])
          n230 = Build Array(w517) -> (w515:string[][])
        }
        frame 61598 {
          # "Ramp Average Current (0xF09E)"
          # "Check"
          n231 = Fract/Exp String To Number(string=w522) -> (number=w521:dbl)  [unwired: 3 in, 1 out]
          n232 = Index Array(array=w526, index=58) -> (element=w528:string)
          n233 = Divide(x=w521, y=1024.0) -> (x/y=w525:dbl)
          n234 = Number To Fractional String(number=w525) -> (F-format string=w524:string)  [unwired: 3 in]
          n235 = Build Array(w528, w524) -> (w527:string[])
          n236 = Build Array(w527) -> (w523:string[][])
        }
        frame 61599 {
          # "Coast Line Voltage (0xF09F)"
          # "Check"
          n237 = Index Array(array=w534, index=59) -> (element=w536:string)
          n238 = call "Q5 Format.vi"("Data (U16 or U32)"=w531) -> ("Q5 Format Data"=w533:string)  [unwired: 10 in]
          n239 = Build Array(w536, w533) -> (w535:string[])
          n240 = Build Array(w535) -> (w532:string[][])
        }
        frame 61600 {
          # "Ramp Speed (0xF0A0)"
          # "Check"
          n241 = Index Array(array=w540, index=60) -> (element=w542:string)
          n242 = Build Array(w542, w538) -> (w541:string[])
          n243 = Build Array(w541) -> (w539:string[][])
        }
        frame 61601 {
          # "Ramp Time (0xF0A1)"
          # "Check"
          n244 = Index Array(array=w546, index=61) -> (element=w548:string)
          n245 = Build Array(w548, w544) -> (w547:string[])
          n246 = Build Array(w547) -> (w545:string[][])
        }
        frame 61602 {
          # "Coast Time (0xF0A2)"
          # "Check"
          n247 = Index Array(array=w552, index=62) -> (element=w554:string)
          n248 = Build Array(w554, w550) -> (w553:string[])
          n249 = Build Array(w553) -> (w551:string[][])
        }
        frame 61603 {
          # "Dry Load Size (0xF0A3)"
          # "Check"
          n250 = Index Array(array=w559, index=63) -> (element=w561:string)
          n251 = call "Q5 Format.vi"("Data (U16 or U32)"=w557) -> ("Q5 Format Data"=w556:string)  [unwired: 10 in]
          n252 = Build Array(w561, w556) -> (w560:string[])
          n253 = Build Array(w560) -> (w558:string[][])
        }
        frame 61604 {
          # "Folding in Acceleration (0xF0A4)"
          # "Check"
          n254 = String Subset(string=w570, offset (0)=0, length (rest)=2 ("length (rest)")) -> (substring=w580:string)
          n255 = String Subset(string=w570, offset (0)=3, length (rest)=2 ("length (rest)")) -> (substring=w579:string)
          n256 = String Subset(string=w570, offset (0)=6, length (rest)=2 ("length (rest)")) -> (substring=w572:string)
          n257 = String Subset(string=w570, offset (0)=9, length (rest)=2 ("length (rest)")) -> (substring=w571:string)
          n258 = Index Array(array=w566, index=64) -> (element=w568:string)
          n259 = Concatenate Strings(w580, w579, w572, w571) -> (w578:string)
          n260 = Hexadecimal String To Number(string=w578) -> (number=w577:u32)  [unwired: 2 in, 1 out]
          n261 = To Long Integer(number=w577) -> (32bit integer=w565:i32)
          n262 = Number To Decimal String(number=w565) -> (decimal integer string=w564:string)  [unwired: 1 in]
          n263 = Build Array(w568, w564) -> (w567:string[])
          n264 = Build Array(w567) -> (w563:string[][])
        }
        frame 61605 {
          # "Max Jerk In Acceleration (0xF0A5)"
          # "Check"
          n265 = String Subset(string=w592, offset (0)=0, length (rest)=2 ("length (rest)")) -> (substring=w602:string)
          n266 = String Subset(string=w592, offset (0)=3, length (rest)=2 ("length (rest)")) -> (substring=w601:string)
          n267 = String Subset(string=w592, offset (0)=6, length (rest)=2 ("length (rest)")) -> (substring=w594:string)
          n268 = String Subset(string=w592, offset (0)=9, length (rest)=2 ("length (rest)")) -> (substring=w593:string)
          n269 = Index Array(array=w586, index=65) -> (element=w590:string)
          n270 = Concatenate Strings(w602, w601, w594, w593) -> (w600:string)
          n271 = Hexadecimal String To Number(string=w600) -> (number=w599:u32)  [unwired: 2 in, 1 out]
          n272 = To Long Integer(number=w599) -> (32bit integer=w588:i32)
          n273 = Number To Decimal String(number=w588) -> (decimal integer string=w587:string)  [unwired: 1 in]
          n274 = Build Array(w590, w587) -> (w589:string[])
          n275 = Build Array(w589) -> (w585:string[][])
        }
        frame 61606 {
          # "Max Jerk In S-S (0xF0A6)"
          # "Check"
          n276 = Index Array(array=w610, index=66) -> (element=w612:string)
          n277 = String Subset(string=w614, offset (0)=0, length (rest)=2 ("length (rest)")) -> (substring=w624:string)
          n278 = String Subset(string=w614, offset (0)=3, length (rest)=2 ("length (rest)")) -> (substring=w623:string)
          n279 = String Subset(string=w614, offset (0)=6, length (rest)=2 ("length (rest)")) -> (substring=w616:string)
          n280 = String Subset(string=w614, offset (0)=9, length (rest)=2 ("length (rest)")) -> (substring=w615:string)
          n281 = Concatenate Strings(w624, w623, w616, w615) -> (w622:string)
          n282 = Hexadecimal String To Number(string=w622) -> (number=w621:u32)  [unwired: 2 in, 1 out]
          n283 = To Long Integer(number=w621) -> (32bit integer=w609:i32)
          n284 = Number To Decimal String(number=w609) -> (decimal integer string=w608:string)  [unwired: 1 in]
          n285 = Build Array(w612, w608) -> (w611:string[])
          n286 = Build Array(w611) -> (w607:string[][])
        }
        frame 61608 {
          # "Shaft Speed (RPM) (0xF0A8)"
          n287 = Index Array(array=w631, index=67) -> (element=w633:string)
          n288 = Build Array(w633, w629) -> (w632:string[])
          n289 = Build Array(w632) -> (w630:string[][])
        }
        frame 61609 {
          # "Basket Speed (RPM) (0xF0A9)"
          # "Check"
          n290 = Index Array(array=w637, index=68) -> (element=w639:string)
          n291 = Build Array(w639, w635) -> (w638:string[])
          n292 = Build Array(w638) -> (w636:string[][])
        }
        frame 61611 {
          # "Current RMS (Amps) (0xF0AB)"
          n293 = Fract/Exp String To Number(string=w642) -> (number=w641:dbl)  [unwired: 3 in, 1 out]
          n294 = Index Array(array=w644, index=69) -> (element=w648:string)
          n295 = Divide(x=w641, y=1024.0) -> (x/y=w646:dbl)
          n296 = Number To Fractional String(number=w646) -> (F-format string=w645:string)  [unwired: 3 in]
          n297 = Build Array(w648, w645) -> (w647:string[])
          n298 = Build Array(w647) -> (w643:string[][])
        }
        frame 61612 {
          # "Target Speed (RPM) (0xF0AC)"
          # "Check"
          n299 = String Subset(string=w658, offset (0)=0, length (rest)=2 ("length (rest)")) -> (substring=w664:string)
          n300 = String Subset(string=w658, offset (0)=3, length (rest)=2 ("length (rest)")) -> (substring=w663:string)
          n301 = Concatenate Strings(w664, w663) -> (w662:string)
          n302 = Hexadecimal String To Number(string=w662) -> (number=w661:u32)  [unwired: 2 in, 1 out]
          n303 = To Word Integer(number=w661) -> (16bit integer=w660:i16)
          n304 = Absolute Value(x=w660) -> (abs(x)=w659:i16)
          n305 = To Unsigned Word Integer(number=w659) -> (unsigned 16bit integer=w654:u16)
          n306 = Number To Decimal String(number=w654) -> (decimal integer string=w653:string)  [unwired: 1 in]
          n307 = Index Array(array=w652, index=70) -> (element=w656:string)
          n308 = Build Array(w656, w653) -> (w655:string[])
          n309 = Build Array(w655) -> (w651:string[][])
        }
        frame 61617 {
          # "Motor Mode (0xF0B1)"
          # "Check"
          n310 = Decimal String To Number(string=w675) -> (number=w676:i32)  [unwired: 2 in, 1 out]
          n311 = Index Array(array=w671, index=71) -> (element=w673:string)
          n312 = case shown="4" w676 {
            tunnel: ["Closed Loop" "Closed Loop Angle" "Open Loop" "Open Loop Angle" "Coasting" "Braking" "Idle"] -> w670
            frame 0, Default {
            }
            frame 1 {
            }
            frame 2 {
            }
            frame 3 {
            }
            frame 4 {
            }
            frame 5 {
            }
            frame 6 {
            }
          }
          n313 = Build Array(w673, w670) -> (w672:string[])
          n314 = Build Array(w672) -> (w669:string[][])
        }
        frame 61619 {
          # "OOB Detected in Acceleration (0xF0B3)"
          # "Check"
          n315 = Index Array(array=w686, index=72) -> (element=w688:string)
          n316 = Build Array(w688, w684) -> (w687:string[])
          n317 = Build Array(w687) -> (w685:string[][])
        }
        frame 61620 {
          # "OOB Detected in S-S (0xF0B4)"
          # "Check"
          n318 = Index Array(array=w692, index=73) -> (element=w694:string)
          n319 = Build Array(w694, w690) -> (w693:string[])
          n320 = Build Array(w693) -> (w691:string[][])
        }
        frame 61621 {
          # "OOB ReDistribution Required (0xF0B5)"
          # "Check"
          n321 = Index Array(array=w698, index=74) -> (element=w700:string)
          n322 = Build Array(w700, w696) -> (w699:string[])
          n323 = Build Array(w699) -> (w697:string[][])
        }
        frame 61623 {
          # "Motor Profile Status (0xF0B7)\nMotor Profile (0xF0B7)"
          # "Check"
          # "Check"
          n324 = String Subset(string=w713, offset (0)=3, length (rest)=2 ("length (rest)")) -> (substring=w718:string)
          n325 = String Subset(string=w713, offset (0)=0, length (rest)=2 ("length (rest)")) -> (substring=w715:string)
          n326 = Index Array(array=w705, index #1=75 ("index"), index #2=76 ("index")) -> (element #1=w710:string, element #2=w709:string)
          n327 = case shown="\"06\"" w718 {
            tunnel: ["Unknown" ("Profile Status") "Started" ("Profile Status") "Stopped" ("Profile Status") "Paused" ("Profile Status") "Resumed" ("Profile Status") "Selected" ("Profile Status") "Completed" ("Profile Status")] -> w704
            frame "00", Default {
            }
            frame "06" {
            }
            frame "07" {
            }
            frame "08" {
            }
            frame "09" {
            }
            frame "0A" {
            }
            frame "0B" {
            }
          }
          n328 = Hexadecimal String To Number(string=w715) -> (number=w714:u32)  [unwired: 2 in, 1 out]
          n329 = Build Array(w710, w709) -> (w708:string[])
          n330 = Number To Decimal String(number=w714) -> (decimal integer string=w703:string)  [unwired: 1 in]
          n331 = Build Array(w704, w703) -> (w707:string[])
          n332 = Build Array(w708, w707) -> (w706:string[][])
          n333 = Transpose 2D Array(2D array=w706) -> (transposed array=w702:string[][])
        }
        frame 65314 {
          # "Mode Shift Status (0xFF22)"
          # "Check"
          n334 = Decimal String To Number(string=w734) -> (number=w735:i32)  [unwired: 2 in, 1 out]
          n335 = Index Array(array=w730, index=77) -> (element=w732:string)
          n336 = case shown="4" w735 {
            tunnel: ["Unknown" ("Motor Profile") "Agitate State" ("Motor Profile") "Spin State" ("Motor Profile") "Trans to Spin" ("Motor Profile") "Trans to Agitate" ("Motor Profile")] -> w729
            frame 0, Default {
            }
            frame 1 {
            }
            frame 2 {
            }
            frame 3 {
            }
            frame 4 {
            }
          }
          n337 = Build Array(w732, w729) -> (w731:string[])
          n338 = Build Array(w731) -> (w728:string[][])
        }
        frame 61630 {
          # "ME Relay (0xF0BE)"
          # "Check"
          n339 = Index Array(array=w743, index=78) -> (element=w745:string)
          n340 = Build Array(w745, w741) -> (w744:string[])
          n341 = Build Array(w744) -> (w742:string[][])
        }
        frame 61631 {
          # "Mode Shift FB (0xF0BF)"
          # "Check"
          n342 = Index Array(array=w749, index=79) -> (element=w751:string)
          n343 = Build Array(w751, w747) -> (w750:string[])
          n344 = Build Array(w750) -> (w748:string[][])
        }
        frame 61632 {
          # "MS Motor (0xF0C0)"
          # "Check"
          n345 = Index Array(array=w755, index=80) -> (element=w757:string)
          n346 = Build Array(w757, w753) -> (w756:string[])
          n347 = Build Array(w756) -> (w754:string[][])
        }
        frame 61636 {
          # "DC Bus Voltage RMS Value (0xF0C4)"
          # "Check"
          n348 = call "Q5 Format.vi"("Data (U16 or U32)"=w765) -> ("Q5 Format Data"=w759:string)  [unwired: 10 in]
          n349 = Index Array(array=w761, index=85) -> (element=w763:string)
          n350 = Build Array(w763, w759) -> (w762:string[])
          n351 = Build Array(w762) -> (w760:string[][])
        }
        frame 61638 {
          # "Partial Coast Time (0xF0C6)"
          # "Check"
          n352 = Index Array(array=w768, index=81) -> (element=w770:string)
          n353 = Build Array(w770, w766) -> (w769:string[])
          n354 = Build Array(w769) -> (w767:string[][])
        }
        frame 61639 {
          # "Ramp Line Voltage (0xF0C7)"
          # "Check"
          n355 = Index Array(array=w775, index=82) -> (element=w777:string)
          n356 = call "Q5 Format.vi"("Data (U16 or U32)"=w773) -> ("Q5 Format Data"=w772:string)  [unwired: 10 in]
          n357 = Build Array(w777, w772) -> (w776:string[])
          n358 = Build Array(w776) -> (w774:string[][])
        }
        frame 65280 {
          # "Personality (0xFF00)"
          n359 = Index Array(array=w781, index=83) -> (element=w783:string)
          n360 = Build Array(w783, w779) -> (w782:string[])
          n361 = Build Array(w782) -> (w780:string[][])
        }
        frame 65282 {
          # "Reset Source (0xFF02)"
          # "Check"
          # "Line Number"
          # "File Name CRC"
          n362 = String Subset(string=w795, offset (0)=0, length (rest)=5 ("length (rest)")) -> (substring=w791:string)
          n363 = String Subset(string=w795, offset (0)=6, length (rest)=2 ("length (rest)")) -> (substring=w800:string)
          n364 = String Subset(string=w795, offset (0)=9, length (rest)=2 ("length (rest)")) -> (substring=w801:string)
          n365 = Concatenate Strings(w800, w801) -> (w802:string)
          n366 = Hexadecimal String To Number(string=w802) -> (number=w793:u32)  [unwired: 2 in, 1 out]
          n367 = Number To Decimal String(number=w793) -> (decimal integer string=w792:string)  [unwired: 1 in]
          n368 = call <vilib>:"Space Constant.vi"() -> ("String"=w794:string)
          n369 = Concatenate Strings(w791, w794, w792) -> (w787:string)
          n370 = Index Array(array=w786, index=84) -> (element=w789:string)
          n371 = Build Array(w789, w787) -> (w788:string[])
          n372 = Build Array(w788) -> (w785:string[][])
        }
      }
    }
    frame "2015 Washer" {
      n373 = case shown="8E" w805 {
        tunnel: w806 -> [_ w830 w831 w854 w856 w857 w863 w869 w875 w887 w900 w912 w926 w940 w953 w961 w979 w985 w992 w1003 w1010 w1016 w1023 w1034 w1045 w1056 w1072 w1086 w1117 w1127 w1140 w1146 w1153 w1168 w1178 w1188 w1197 w1213 w1223 w1228 w1238 w1248 w1258 w1268 w1290 w1304 w1305 w1312 w1322 w1331 w1338 w1344 w1350 w1357 w1370 w1392 w1414 w1429 w1435 w1442 w1458 w1475 w1484 w1490 w1496 w1513 w1534 w1541 w1547 w1553 w1565 w1566 w1573 w1579 w1595]
        tunnel: [string[][] [] w810 w832 w837 string[][] [] w858 w864 w870 w876 w881 w894 w906 w920 w934 w947 w955 w980 w986 w991 w997 w1011 w1017 w1028 w1035 w1046 w1057 w1066 w1088 w1092 w1120 w1134 w1147 w1154 w1162 w1172 w1182 w1198 w1207 w1217 w1229 w1239 w1249 w1259 w1269 w1277 w1291 w1307 w1315 w1323 w1332 w1339 w1345 w1351 w1358 w1363 w1385 w1407 w1430 w1436 w1443 w1451 w1469 w1485 w1491 w1497 w1502 w1528 w1542 w1548 w1554 w1560 w1567 w1574 w1580 w1585] -> w808
        tunnel: w807 -> [_ w812 w836 w853 _ w862 w868 w871 w877 w883 w896 w907 w922 w936 w949 w957 w981 w987 w993 w999 w1012 w1018 w1029 w1036 w1047 w1059 w1068 w1089 w1097 w1123 w1135 w1148 w1157 w1163 w1174 w1184 w1202 w1208 w1219 w1232 w1242 w1250 w1260 w1272 w1282 w1296 w1306 w1316 w1326 w1334 w1340 w1346 w1352 w1359 w1366 w1386 w1410 w1431 w1437 w1444 w1452 w1471 w1486 w1492 w1498 w1505 w1530 w1543 w1549 w1555 w1561 w1568 w1575 w1581 w1586]
        frame Default {
        }
        frame 256 {
          # "Critical Major (0x0100)\nCritical Minor (0x0100)\nNon-Critical Major (0x0100)\nNon-Critical Minor (0x0100)\nDaily Revision (0x0100)"
          # "Check"
          n374 = Index Array(array=w812, index #1=0 ("index"), index #2=1 ("index"), index #3=2 ("index"), index #4=3 ("index"), index #5=4 ("index")) -> (element #1=w824:string, element #2=w823:string, element #3=w822:string, element #4=w821:string, element #5=w820:string)
          n375 = Build Array(w824, w823, w822, w821, w820) -> (w814:string[])
          n376 = call "Get Software Version.vi"("Data"=w830) -> ("Daily Revision"=w815:string, "Non-Critical Major"=w817:string, "Critical Minor"=w818:string, "Critical Major"=w819:string, "Non-Critical Minor"=w816:string)  [unwired: 6 in]
          n377 = Build Array(w819, w818, w817, w816, w815) -> (w813:string[])
          n378 = Build Array(w814, w813) -> (w811:string[][])
          n379 = Transpose 2D Array(2D array=w811) -> (transposed array=w810:string[][])
        }
        frame 142 {
          # "Cycle Count (0x008E)"
          # "Check"
          n380 = Index Array(array=w836, index=5) -> (element=w834:string)
          n381 = Build Array(w834, w831) -> (w833:string[])
          n382 = Build Array(w833) -> (w832:string[][])
        }
        frame 61441 {
          # "XML Critical Major (0xF001)\nXML Critical Minor (0xF001)\nXML Non-Critical Major (0xF001)\nXML Non-Critical Minor (0xF001)"
          # "Check"
          n383 = Index Array(array=w853, index #1=6 ("index"), index #2=7 ("index"), index #3=8 ("index"), index #4=9 ("index")) -> (element #1=w848:string, element #2=w847:string, element #3=w846:string, element #4=w845:string)
          n384 = Build Array(w848, w847, w846, w845) -> (w840:string[])
          n385 = call "XML Version.vi"("Data"=w854) -> ("XML Non-Critical Minor"=w841:string, "XML Non-Critical Major"=w842:string, "XML Critical Minor"=w843:string, "XML Critical Major"=w844:string)  [unwired: 7 in]
          n386 = Build Array(w844, w843, w842, w841) -> (w839:string[])
          n387 = Build Array(w840, w839) -> (w838:string[][])
          n388 = Transpose 2D Array(2D array=w838) -> (transposed array=w837:string[][])
        }
        frame 61457 {
          # "Skipping this one"
          # "Check"
          n389 = call "Red_Micro_Parse.vi"("Data"=w856) -> ()  [unwired: 10 in, 1 out]
        }
        frame 61460 {
          # "Available Free Stack % (0xF014)"
          n390 = Index Array(array=w862, index=10) -> (element=w860:string)
          n391 = Build Array(w860, w857) -> (w859:string[])
          n392 = Build Array(w859) -> (w858:string[][])
        }
        frame 61697 {
          # "Extra Rinse (0xF101)"
          # "Check"
          n393 = Index Array(array=w868, index=11) -> (element=w866:string)
          n394 = Build Array(w866, w863) -> (w865:string[])
          n395 = Build Array(w865) -> (w864:string[][])
        }
        frame 61698 {
          # "Deep Rinse_Fabric Softener (0xF102)"
          # "Check"
          n396 = Index Array(array=w871, index=12) -> (element=w873:string)
          n397 = Build Array(w873, w869) -> (w872:string[])
          n398 = Build Array(w872) -> (w870:string[][])
        }
        frame 61699 {
          # "My Cycle (0xF103)"
          # "Check"
          n399 = Index Array(array=w877, index=13) -> (element=w879:string)
          n400 = Build Array(w879, w875) -> (w878:string[])
          n401 = Build Array(w878) -> (w876:string[][])
        }
        frame 61749 {
          # "Soil Level (0xF135)"
          # "Check"
          n402 = case shown="\"04\"" w887 {
            selector: w887 -> [w888 _ _ _ _ _]
            tunnel: [w888 "EXTRA LIGHT" "LIGHT" "NORMAL" "HEAVY" "EXTRA HEAVY"] -> w882
            frame Default {
            }
            frame "00" {
            }
            frame "01" {
            }
            frame "02" {
            }
            frame "03" {
            }
            frame "04" {
            }
          }
          n403 = Index Array(array=w883, index=14) -> (element=w885:string)
          n404 = Build Array(w885, w882) -> (w884:string[])
          n405 = Build Array(w884) -> (w881:string[][])
        }
        frame 61752 {
          # "Spin Level (0xF138)"
          # "Check"
          n406 = case shown="\"03\"" w900 {
            selector: w900 -> [w901 _ _ _ _]
            tunnel: [w901 "NO SPIN" "NORMAL" "MORE " "MAX"] -> w895
            frame Default {
            }
            frame "00" {
            }
            frame "01" {
            }
            frame "02" {
            }
            frame "03" {
            }
          }
          n407 = Index Array(array=w896, index=15) -> (element=w898:string)
          n408 = Build Array(w898, w895) -> (w897:string[])
          n409 = Build Array(w897) -> (w894:string[][])
        }
        frame 61751 {
          # "Stain (0xF137)"
          # "Check"
          n410 = case shown="\"01\"" w912 {
            selector: w912 -> [w913 _ _ _ _ _ _]
            tunnel: [w913 "OFF" "TOMATO" "WINE" "BLOOD" "GRASS" "DIRT"] -> w908
            frame Default {
            }
            frame "00" {
            }
            frame "01" {
            }
            frame "02" {
            }
            frame "03" {
            }
            frame "04" {
            }
            frame "05" {
            }
          }
          n411 = Index Array(array=w907, index=16) -> (element=w910:string)
          n412 = Build Array(w910, w908) -> (w909:string[])
          n413 = Build Array(w909) -> (w906:string[][])
        }
        frame 61750 {
          # "Temperature Level (0xF136)"
          n414 = case shown="\"05\"" w926 {
            selector: w926 -> [w927 _ _ _ _ _ _]
            tunnel: [w927 "TAP COLD" "COLD" "COOL" "COLORS" "WARM" "HOT"] -> w921
            frame Default {
            }
            frame "00" {
            }
            frame "01" {
            }
            frame "02" {
            }
            frame "03" {
            }
            frame "04" {
            }
            frame "05" {
            }
          }
          n415 = Index Array(array=w922, index=17) -> (element=w924:string)
          n416 = Build Array(w924, w921) -> (w923:string[])
          n417 = Build Array(w923) -> (w920:string[][])
        }
        frame 61748 {
          # "Load Size (0xF134)"
          # "Check"
          n418 = case shown="\"04\"" w940 {
            selector: w940 -> [w941 _ _ _ _ _]
            tunnel: [w941 "SMALL" "MEDIUM" "LARGE" "SUPER" "PRECISE FILL"] -> w935
            frame Default {
            }
            frame "00" {
            }
            frame "01" {
            }
            frame "02" {
            }
            frame "03" {
            }
            frame "04" {
            }
          }
          n419 = Index Array(array=w936, index=18) -> (element=w938:string)
          n420 = Build Array(w938, w935) -> (w937:string[])
          n421 = Build Array(w937) -> (w934:string[][])
        }
        frame 61706 {
          # "Machine State (0xF10A)"
          # "Check"
          n422 = Decimal String To Number(string=w953) -> (number=w954:i32)  [unwired: 2 in, 1 out]
          n423 = Index Array(array=w949, index=19) -> (element=w951:string)
          n424 = call "Machine State.vi"("Numeric"=w954) -> ("Profile Status"=w948:string)  [unwired: 10 in]
          n425 = Build Array(w951, w948) -> (w950:string[])
          n426 = Build Array(w950) -> (w947:string[][])
        }
        frame 61708 {
          # "Cycle Selected (0xF10C)"
          # "Check"
          n427 = Decimal String To Number(string=w961) -> (number=w962:i32)  [unwired: 2 in, 1 out]
          n428 = Index Array(array=w957, index=20) -> (element=w959:string)
          n429 = case shown="6" w962 {
            tunnel: ["Cycle 0" ("Motor Profile") "Cycle 1" ("Motor Profile") "Cycle 2" ("Motor Profile") "Cycle 3" ("Motor Profile") "Cycle 4" ("Motor Profile") "Cycle 5" ("Motor Profile") "Cycle 6" ("Motor Profile") "Cycle 7" ("Motor Profile") "Cycle 8" ("Motor Profile") "Cycle 9" ("Motor Profile") "Cycle 10" ("Motor Profile") "Cycle 11" ("Motor Profile") "Cycle 12" ("Motor Profile") "Cycle 13" ("Motor Profile") "Cycle 14" ("Motor Profile") "Cycle 15" ("Motor Profile")] -> w956
            frame 0, Default {
            }
            frame 1 {
            }
            frame 2 {
            }
            frame 3 {
            }
            frame 4 {
            }
            frame 5 {
            }
            frame 6 {
            }
            frame 7 {
            }
            frame 8 {
            }
            frame 9 {
            }
            frame 10 {
            }
            frame 11 {
            }
            frame 12 {
            }
            frame 13 {
            }
            frame 14 {
            }
            frame 15 {
            }
          }
          n430 = Build Array(w959, w956) -> (w958:string[])
          n431 = Build Array(w958) -> (w955:string[][])
        }
        frame 61709 {
          # "Delay Time (0xF10D)"
          # "Might not work"
          n432 = Index Array(array=w981, index=21) -> (element=w983:string)
          n433 = Build Array(w983, w979) -> (w982:string[])
          n434 = Build Array(w982) -> (w980:string[][])
        }
        frame 61710 {
          # "Soak Time (0xF10E)"
          # "Check"
          n435 = Index Array(array=w987, index=22) -> (element=w989:string)
          n436 = Build Array(w989, w985) -> (w988:string[])
          n437 = Build Array(w988) -> (w986:string[][])
        }
        frame 61726 {
          # "Auto Soak Level (0xF11E)"
          # "Check"
          n438 = Index Array(array=w993, index=23) -> (element=w995:string)
          n439 = Build Array(w995, w992) -> (w994:string[])
          n440 = Build Array(w994) -> (w991:string[][])
        }
        frame 61731 {
          # "Deep Fill (0xF123)"
          # "Check. Could add names:\n00=Off\n01=Incremental Fill\n02=Max Fill"
          n441 = case shown="\"00\", Default" w1003 {
            tunnel: [FALSE ("Eco Wash") TRUE ("Eco Wash") TRUE ("Eco Wash")] -> _
            tunnel: ["Off" "Incremental Fill" "Max Fill"] -> w998
            frame "00", Default {
            }
            frame "01" {
            }
            frame "02" {
            }
          }
          n442 = Index Array(array=w999, index=24) -> (element=w1001:string)
          n443 = Build Array(w1001, w998) -> (w1000:string[])
          n444 = Build Array(w1000) -> (w997:string[][])
        }
        frame 61732 {
          # "Warm Rinse (0xF124)"
          # "Check"
          n445 = Index Array(array=w1012, index=25) -> (element=w1014:string)
          n446 = Build Array(w1014, w1010) -> (w1013:string[])
          n447 = Build Array(w1013) -> (w1011:string[][])
        }
        frame 61760 {
          # "Remaining Cycle Time(s) (0xF140)"
          # "Check"
          n448 = Index Array(array=w1018, index=26) -> (element=w1020:string)
          n449 = Build Array(w1020, w1016) -> (w1019:string[])
          n450 = Build Array(w1019) -> (w1017:string[][])
        }
        frame 61952 {
          # "Wet Load Gallons (0xF200)"
          # "Check"
          n451 = Fract/Exp String To Number(string=w1023) -> (number=w1022:dbl)  [unwired: 3 in, 1 out]
          n452 = Index Array(array=w1029, index=27) -> (element=w1031:string)
          n453 = Divide(x=w1022, y=100.0) -> (x/y=w1027:dbl)
          n454 = Number To Fractional String(number=w1027, precision (6)=i16 3) -> (F-format string=w1024:string)  [unwired: 2 in]
          n455 = Build Array(w1031, w1024) -> (w1030:string[])
          n456 = Build Array(w1030) -> (w1028:string[][])
        }
        frame 61953 {
          # "Tub Volume Gallons (0xF201)"
          # "Check"
          n457 = Fract/Exp String To Number(string=w1034) -> (number=w1033:dbl)  [unwired: 3 in, 1 out]
          n458 = Index Array(array=w1036, index=28) -> (element=w1041:string)
          n459 = Divide(x=w1033, y=100.0) -> (x/y=w1037:dbl)
          n460 = Number To Fractional String(number=w1037, precision (6)=i16 3) -> (F-format string=w1038:string)  [unwired: 2 in]
          n461 = Build Array(w1041, w1038) -> (w1040:string[])
          n462 = Build Array(w1040) -> (w1035:string[][])
        }
        frame 61954 {
          # "Pressure (inches of H20) (0xF202)"
          n463 = Fract/Exp String To Number(string=w1045) -> (number=w1044:dbl)  [unwired: 3 in, 1 out]
          n464 = Index Array(array=w1047, index=29) -> (element=w1052:string)
          n465 = Divide(x=w1044, y=1000.0) -> (x/y=w1048:dbl)
          n466 = Number To Fractional String(number=w1048, precision (6)=i16 3) -> (F-format string=w1049:string)  [unwired: 2 in]
          n467 = Build Array(w1052, w1049) -> (w1051:string[])
          n468 = Build Array(w1051) -> (w1046:string[][])
        }
        frame 61957 {
          # "Target Gallons (0xF205)"
          # "Check"
          n469 = Fract/Exp String To Number(string=w1056) -> (number=w1055:dbl)  [unwired: 3 in, 1 out]
          n470 = Index Array(array=w1059, index=30) -> (element=w1063:string)
          n471 = Divide(x=w1055, y=100.0) -> (x/y=w1058:dbl)
          n472 = Number To Fractional String(number=w1058, precision (6)=i16 3) -> (F-format string=w1060:string)  [unwired: 2 in]
          n473 = Build Array(w1063, w1060) -> (w1062:string[])
          n474 = Build Array(w1062) -> (w1057:string[][])
        }
        frame 61958 {
          # "Load Type (0xF206)"
          # "Check....could use the U8 conversion"
          n475 = case shown="\"3\"" w1072 {
            selector: w1072 -> [w1073 _ _ _ _ _ _ _ _ _ _ _ _]
            tunnel: [w1073 "UNKNOWN" "COTTON" "SYNTHETIC" "MIXED" "WET" "LOW FLOW" "SMALL" "MEDIUM" "LARGE" "SUPER" "SUPER PLUS" "MAX"] -> w1067
            frame Default {
            }
            frame "0" {
            }
            frame "1" {
            }
            frame "2" {
            }
            frame "3" {
            }
            frame "4" {
            }
            frame "5" {
            }
            frame "6" {
            }
            frame "7" {
            }
            frame "8" {
            }
            frame "9" {
            }
            frame "10" {
            }
            frame "11" {
            }
          }
          n476 = Index Array(array=w1068, index=31) -> (element=w1070:string)
          n477 = Build Array(w1070, w1067) -> (w1069:string[])
          n478 = Build Array(w1069) -> (w1066:string[][])
        }
        frame 61959 {
          # "Lid Switch (0xF207)"
          # "Check"
          n479 = Index Array(array=w1089, index=32) -> (element=w1091:string)
          n480 = Build Array(w1091, w1086) -> (w1090:string[])
          n481 = Build Array(w1090) -> (w1088:string[][])
        }
        frame 61961 {
          # "Hot Water Valve (0xF209)\nCold Water Valve (0xF209)\nSpray_Rinse Valve (0xF209)\nFabric Softener Valve (0xF209)"
          # "Check"
          n482 = Index Array(array=w1097, index #1=33 ("index"), index #2=34 ("index"), index #3=35 ("index"), index #4=36 ("index")) -> (element #1=w1104:string, element #2=w1103:string, element #3=w1102:string, element #4=w1101:string)
          n483 = Build Array(w1104, w1103, w1102, w1101) -> (w1100:string[])
          n484 = Decimal String To Number(string=w1117) -> (number=w1118:i32)  [unwired: 2 in, 1 out]
          n485 = Number To Boolean Array(number=w1118) -> (Boolean array=w1119:bool[])
          n486 = Index Array(array=w1119) -> (element #1=w1112:bool, element #2=w1111:bool, element #3=w1110:bool, element #4=w1109:bool)  [unwired: 4 in]
          n487 = Boolean To (0,1)(Boolean=w1112) -> (0, 1=w1116:i16)
          n488 = Boolean To (0,1)(Boolean=w1111) -> (0, 1=w1115:i16)
          n489 = Boolean To (0,1)(Boolean=w1110) -> (0, 1=w1114:i16)
          n490 = Boolean To (0,1)(Boolean=w1109) -> (0, 1=w1113:i16)
          n491 = Number To Decimal String(number=w1116) -> (decimal integer string=w1096:string)  [unwired: 1 in]
          n492 = Number To Decimal String(number=w1115) -> (decimal integer string=w1095:string)  [unwired: 1 in]
          n493 = Number To Decimal String(number=w1114) -> (decimal integer string=w1094:string)  [unwired: 1 in]
          n494 = Number To Decimal String(number=w1113) -> (decimal integer string=w1093:string)  [unwired: 1 in]
          n495 = Build Array(w1096, w1095, w1094, w1093) -> (w1099:string[])
          n496 = Build Array(w1100, w1099) -> (w1098:string[][])
          n497 = Transpose 2D Array(2D array=w1098) -> (transposed array=w1092:string[][])
        }
        frame 61962 {
          # "Lid Lock Req State (0xF20A)"
          # "Check"
          n498 = String Subset(string=w1127, offset (0)=3, length (rest)=2 ("length (rest)")) -> (substring=w1128:string)
          n499 = Index Array(array=w1123, index=37) -> (element=w1125:string)
          n500 = Hexadecimal String To Number(string=w1128) -> (number=w1126:u32)  [unwired: 2 in, 1 out]
          n501 = case shown="0, Default" w1126 {
            tunnel: ["UNLOCKED" "LOCKED" "FAILURE"] -> w1121
            frame 0, Default {
            }
            frame 1 {
            }
            frame 2 {
            }
          }
          n502 = Build Array(w1125, w1121) -> (w1124:string[])
          n503 = Build Array(w1124) -> (w1120:string[][])
        }
        frame 61963 {
          # "Lid Lock Status (0xF20B)"
          # "Check"
          n504 = Decimal String To Number(string=w1140) -> (number=w1141:i32)  [unwired: 2 in, 1 out]
          n505 = Index Array(array=w1135, index=38) -> (element=w1138:string)
          n506 = case shown="2" w1141 {
            tunnel: ["Unlocked" ("Motor Profile") "Locked" ("Motor Profile") "Failure" ("Motor Profile")] -> w1136
            frame 0, Default {
            }
            frame 1 {
            }
            frame 2 {
            }
          }
          n507 = Build Array(w1138, w1136) -> (w1137:string[])
          n508 = Build Array(w1137) -> (w1134:string[][])
        }
        frame 61964 {
          # "Cycle Engine State (0xF20C)"
          n509 = call "Cycle Engine State.vi"("Data"=w1146) -> ("Cycle Engine State"=w1145:string)  [unwired: 10 in]
          n510 = Index Array(array=w1148, index=39) -> (element=w1150:string)
          n511 = Build Array(w1150, w1145) -> (w1149:string[])
          n512 = Build Array(w1149) -> (w1147:string[][])
        }
        frame 61967 {
          # "Current Water Temperature (°F) (0xF20F)"
          # "Check"
          n513 = Fract/Exp String To Number(string=w1153) -> (number=w1152:dbl)  [unwired: 3 in, 1 out]
          n514 = Index Array(array=w1157, index=40) -> (element=w1159:string)
          n515 = Divide(x=w1152, y=10.0) -> (x/y=w1156:dbl)
          n516 = Number To Fractional String(number=w1156) -> (F-format string=w1155:string)  [unwired: 3 in]
          n517 = Build Array(w1159, w1155) -> (w1158:string[])
          n518 = Build Array(w1158) -> (w1154:string[][])
        }
        frame 61968 {
          # "Drain Pump (0xF210)"
          # "Check"
          n519 = String Subset(string=w1168, offset (0)=3, length (rest)=2 ("length (rest)")) -> (substring=w1169:string)
          n520 = Index Array(array=w1163, index=41) -> (element=w1166:string)
          n521 = call "HexStringToBoolean.vi"("Hex String"=w1169) -> ("decimal integer string"=w1164:string)  [unwired: 1 in, 1 out]
          n522 = Build Array(w1166, w1164) -> (w1165:string[])
          n523 = Build Array(w1165) -> (w1162:string[][])
        }
        frame 61969 {
          # "Recirculating Pump (0xF211)"
          n524 = String Subset(string=w1178, offset (0)=3, length (rest)=2 ("length (rest)")) -> (substring=w1179:string)
          n525 = Index Array(array=w1174, index=42) -> (element=w1176:string)
          n526 = call "HexStringToBoolean.vi"("Hex String"=w1179) -> ("decimal integer string"=w1173:string)  [unwired: 1 in, 1 out]
          n527 = Build Array(w1176, w1173) -> (w1175:string[])
          n528 = Build Array(w1175) -> (w1172:string[][])
        }
        frame 61971 {
          # "Sub-Cycle (0xF213)"
          # "Check"
          n529 = case shown="\"04\"" w1188 {
            selector: w1188 -> [w1189 _ _ _ _ _ _]
            tunnel: [w1189 "NONE" "FILL" "SOAK" "WASH" "RINSE" "SPIN"] -> w1183
            frame Default {
            }
            frame "00" {
            }
            frame "01" {
            }
            frame "02" {
            }
            frame "04" {
            }
            frame "08" {
            }
            frame "10" {
            }
          }
          n530 = Index Array(array=w1184, index=43) -> (element=w1186:string)
          n531 = Build Array(w1186, w1183) -> (w1185:string[])
          n532 = Build Array(w1185) -> (w1182:string[][])
        }
        frame 61973 {
          # "Target Level Inches (0xF215)"
          # "Check"
          n533 = Fract/Exp String To Number(string=w1197) -> (number=w1196:dbl)  [unwired: 3 in, 1 out]
          n534 = Index Array(array=w1202, index=44) -> (element=w1204:string)
          n535 = Divide(x=w1196, y=1000.0) -> (x/y=w1201:dbl)
          n536 = Number To Fractional String(number=w1201, precision (6)=i16 3) -> (F-format string=w1199:string)  [unwired: 2 in]
          n537 = Build Array(w1204, w1199) -> (w1203:string[])
          n538 = Build Array(w1203) -> (w1198:string[][])
        }
        frame 61976 {
          # "Valve Relay (0xF218)"
          # "Check"
          n539 = String Subset(string=w1213, offset (0)=3, length (rest)=2 ("length (rest)")) -> (substring=w1214:string)
          n540 = Index Array(array=w1208, index=45) -> (element=w1211:string)
          n541 = call "HexStringToBoolean.vi"("Hex String"=w1214) -> ("decimal integer string"=w1209:string)  [unwired: 1 in, 1 out]
          n542 = Build Array(w1211, w1209) -> (w1210:string[])
          n543 = Build Array(w1210) -> (w1207:string[][])
        }
        frame 61977 {
          # "Lid Lock FB (0xF219)"
          # "Check"
          n544 = case shown="\"01\"" w1223 {
            selector: w1223 -> [w1224 _ _]
            tunnel: [w1224 "LOCKED" ("Motor Profile") "UNLOCKED" ("Motor Profile")] -> w1218
            frame "0", Default {
            }
            frame "00" {
            }
            frame "01" {
            }
          }
          n545 = Index Array(array=w1219, index=46) -> (element=w1221:string)
          n546 = Build Array(w1221, w1218) -> (w1220:string[])
          n547 = Build Array(w1220) -> (w1217:string[][])
        }
        frame 61985 {
          # "Target Bath Temperature (°F) (0xF221)"
          # "Check"
          n548 = Fract/Exp String To Number(string=w1228) -> (number=w1227:dbl)  [unwired: 3 in, 1 out]
          n549 = Index Array(array=w1232, index=47) -> (element=w1234:string)
          n550 = Divide(x=w1227, y=10.0) -> (x/y=w1231:dbl)
          n551 = Number To Fractional String(number=w1231) -> (F-format string=w1230:string)  [unwired: 3 in]
          n552 = Build Array(w1234, w1230) -> (w1233:string[])
          n553 = Build Array(w1233) -> (w1229:string[][])
        }
        frame 61986 {
          # "Current Bath Temperature (°F) (0xF222)"
          # "Check"
          n554 = Fract/Exp String To Number(string=w1238) -> (number=w1237:dbl)  [unwired: 3 in, 1 out]
          n555 = Index Array(array=w1242, index=48) -> (element=w1244:string)
          n556 = Divide(x=w1237, y=10.0) -> (x/y=w1241:dbl)
          n557 = Number To Fractional String(number=w1241) -> (F-format string=w1240:string)  [unwired: 3 in]
          n558 = Build Array(w1244, w1240) -> (w1243:string[])
          n559 = Build Array(w1243) -> (w1239:string[][])
        }
        frame 61987 {
          # "Cold Inlet Temperature (°F) (0xF223)"
          # "Check"
          n560 = Fract/Exp String To Number(string=w1248) -> (number=w1247:dbl)  [unwired: 3 in, 1 out]
          n561 = Index Array(array=w1250, index=49) -> (element=w1254:string)
          n562 = Divide(x=w1247, y=10.0) -> (x/y=w1252:dbl)
          n563 = Number To Fractional String(number=w1252) -> (F-format string=w1251:string)  [unwired: 3 in]
          n564 = Build Array(w1254, w1251) -> (w1253:string[])
          n565 = Build Array(w1253) -> (w1249:string[][])
        }
        frame 61988 {
          # "Hot Inlet Temperature (°F) (0xF224)"
          # "Check"
          n566 = Fract/Exp String To Number(string=w1258) -> (number=w1257:dbl)  [unwired: 3 in, 1 out]
          n567 = Index Array(array=w1260, index=50) -> (element=w1264:string)
          n568 = Divide(x=w1257, y=10.0) -> (x/y=w1262:dbl)
          n569 = Number To Fractional String(number=w1262) -> (F-format string=w1261:string)  [unwired: 3 in]
          n570 = Build Array(w1264, w1261) -> (w1263:string[])
          n571 = Build Array(w1263) -> (w1259:string[][])
        }
        frame 61989 {
          # "Warm Inlet Temperature (°F) (0xF225)"
          # "Check"
          n572 = Fract/Exp String To Number(string=w1268) -> (number=w1267:dbl)  [unwired: 3 in, 1 out]
          n573 = Index Array(array=w1272, index=51) -> (element=w1274:string)
          n574 = Divide(x=w1267, y=10.0) -> (x/y=w1271:dbl)
          n575 = Number To Fractional String(number=w1271) -> (F-format string=w1270:string)  [unwired: 3 in]
          n576 = Build Array(w1274, w1270) -> (w1273:string[])
          n577 = Build Array(w1273) -> (w1269:string[][])
        }
        frame 61990 {
          # "Hot Gallons (0xF226)\nCold Gallons (0xF226)"
          # "Check"
          # "Check"
          n578 = call "Hot and Cold Gallons.vi"("Data"=w1290) -> ("ColdGallons"=w1280:dbl, "Hot Gallons"=w1281:dbl)  [unwired: 9 in]
          n579 = Index Array(array=w1282, index #1=52 ("index"), index #2=53 ("index")) -> (element #1=w1287:string, element #2=w1286:string)
          n580 = Number To Fractional String(number=w1281) -> (F-format string=w1279:string)  [unwired: 3 in]
          n581 = Number To Fractional String(number=w1280) -> (F-format string=w1278:string)  [unwired: 3 in]
          n582 = Build Array(w1287, w1286) -> (w1285:string[])
          n583 = Build Array(w1279, w1278) -> (w1284:string[])
          n584 = Build Array(w1285, w1284) -> (w1283:string[][])
          n585 = Transpose 2D Array(2D array=w1283) -> (transposed array=w1277:string[][])
        }
        frame 61991 {
          # "Hot Seg Valve Time (0xF227)\nCold Seg Valve Time (0xF227)"
          # "Check"
          # "Check"
          n586 = Index Array(array=w1296, index #1=54 ("index"), index #2=55 ("index")) -> (element #1=w1301:string, element #2=w1300:string)
          n587 = Build Array(w1301, w1300) -> (w1299:string[])
          n588 = call "Segment Valve Time.vi"("Data"=w1304) -> ("Cold Segment Valve Time"=w1292:u16, "Hot Segment Valve Time"=w1293:u16)  [unwired: 9 in]
          n589 = Number To Decimal String(number=w1293) -> (decimal integer string=w1295:string)  [unwired: 1 in]
          n590 = Number To Decimal String(number=w1292) -> (decimal integer string=w1294:string)  [unwired: 1 in]
          n591 = Build Array(w1295, w1294) -> (w1298:string[])
          n592 = Build Array(w1299, w1298) -> (w1297:string[][])
          n593 = Transpose 2D Array(2D array=w1297) -> (transposed array=w1291:string[][])
        }
        frame 61994 {
          # "Child Safety (0xF22A)"
          # "Check"
          n594 = Index Array(array=w1306, index=56) -> (element=w1309:string)
          n595 = Build Array(w1309, w1305) -> (w1308:string[])
          n596 = Build Array(w1308) -> (w1307:string[][])
        }
        frame 61995 {
          # "Segment Gallons (0xF22B)"
          # "Check"
          n597 = Fract/Exp String To Number(string=w1312) -> (number=w1311:dbl)  [unwired: 3 in, 1 out]
          n598 = Index Array(array=w1316, index=57) -> (element=w1318:string)
          n599 = Divide(x=w1311, y=100.0) -> (x/y=w1314:dbl)
          n600 = Number To Fractional String(number=w1314) -> (F-format string=w1313:string)  [unwired: 3 in]
          n601 = Build Array(w1318, w1313) -> (w1317:string[])
          n602 = Build Array(w1317) -> (w1315:string[][])
        }
        frame 62208 {
          # "Ramp Average Current (0xF300)"
          # "Check"
          n603 = Fract/Exp String To Number(string=w1322) -> (number=w1321:dbl)  [unwired: 3 in, 1 out]
          n604 = Index Array(array=w1326, index=58) -> (element=w1328:string)
          n605 = Divide(x=w1321, y=1024.0) -> (x/y=w1325:dbl)
          n606 = Number To Fractional String(number=w1325) -> (F-format string=w1324:string)  [unwired: 3 in]
          n607 = Build Array(w1328, w1324) -> (w1327:string[])
          n608 = Build Array(w1327) -> (w1323:string[][])
        }
        frame 62209 {
          # "Coast Line Voltage (0xF301)"
          # "Check"
          n609 = Index Array(array=w1334, index=59) -> (element=w1336:string)
          n610 = call "Q5 Format.vi"("Data (U16 or U32)"=w1331) -> ("Q5 Format Data"=w1333:string)  [unwired: 10 in]
          n611 = Build Array(w1336, w1333) -> (w1335:string[])
          n612 = Build Array(w1335) -> (w1332:string[][])
        }
        frame 62210 {
          # "Ramp Speed (0xF302)"
          # "Check"
          n613 = Index Array(array=w1340, index=60) -> (element=w1342:string)
          n614 = Build Array(w1342, w1338) -> (w1341:string[])
          n615 = Build Array(w1341) -> (w1339:string[][])
        }
        frame 62211 {
          # "Ramp Time (0xF303)"
          # "Check"
          n616 = Index Array(array=w1346, index=61) -> (element=w1348:string)
          n617 = Build Array(w1348, w1344) -> (w1347:string[])
          n618 = Build Array(w1347) -> (w1345:string[][])
        }
        frame 62212 {
          # "Coast Time (0xF304)"
          # "Check"
          n619 = Index Array(array=w1352, index=62) -> (element=w1354:string)
          n620 = Build Array(w1354, w1350) -> (w1353:string[])
          n621 = Build Array(w1353) -> (w1351:string[][])
        }
        frame 62213 {
          # "Dry Load Size (0xF305)"
          # "Check"
          n622 = Index Array(array=w1359, index=63) -> (element=w1361:string)
          n623 = call "Q5 Format.vi"("Data (U16 or U32)"=w1357) -> ("Q5 Format Data"=w1356:string)  [unwired: 10 in]
          n624 = Build Array(w1361, w1356) -> (w1360:string[])
          n625 = Build Array(w1360) -> (w1358:string[][])
        }
        frame 62214 {
          # "Folding in Acceleration (0xF306)"
          # "Check"
          n626 = String Subset(string=w1370, offset (0)=0, length (rest)=2 ("length (rest)")) -> (substring=w1380:string)
          n627 = String Subset(string=w1370, offset (0)=3, length (rest)=2 ("length (rest)")) -> (substring=w1379:string)
          n628 = String Subset(string=w1370, offset (0)=6, length (rest)=2 ("length (rest)")) -> (substring=w1372:string)
          n629 = String Subset(string=w1370, offset (0)=9, length (rest)=2 ("length (rest)")) -> (substring=w1371:string)
          n630 = Index Array(array=w1366, index=64) -> (element=w1368:string)
          n631 = Concatenate Strings(w1380, w1379, w1372, w1371) -> (w1378:string)
          n632 = Hexadecimal String To Number(string=w1378) -> (number=w1377:u32)  [unwired: 2 in, 1 out]
          n633 = To Long Integer(number=w1377) -> (32bit integer=w1365:i32)
          n634 = Number To Decimal String(number=w1365) -> (decimal integer string=w1364:string)  [unwired: 1 in]
          n635 = Build Array(w1368, w1364) -> (w1367:string[])
          n636 = Build Array(w1367) -> (w1363:string[][])
        }
        frame 62215 {
          # "Max Jerk In Acceleration (0xF307)"
          # "Check"
          n637 = String Subset(string=w1392, offset (0)=0, length (rest)=2 ("length (rest)")) -> (substring=w1402:string)
          n638 = String Subset(string=w1392, offset (0)=3, length (rest)=2 ("length (rest)")) -> (substring=w1401:string)
          n639 = String Subset(string=w1392, offset (0)=6, length (rest)=2 ("length (rest)")) -> (substring=w1394:string)
          n640 = String Subset(string=w1392, offset (0)=9, length (rest)=2 ("length (rest)")) -> (substring=w1393:string)
          n641 = Index Array(array=w1386, index=65) -> (element=w1390:string)
          n642 = Concatenate Strings(w1402, w1401, w1394, w1393) -> (w1400:string)
          n643 = Hexadecimal String To Number(string=w1400) -> (number=w1399:u32)  [unwired: 2 in, 1 out]
          n644 = To Long Integer(number=w1399) -> (32bit integer=w1388:i32)
          n645 = Number To Decimal String(number=w1388) -> (decimal integer string=w1387:string)  [unwired: 1 in]
          n646 = Build Array(w1390, w1387) -> (w1389:string[])
          n647 = Build Array(w1389) -> (w1385:string[][])
        }
        frame 62216 {
          # "Max Jerk In S-S (0xF308)"
          # "Check"
          n648 = String Subset(string=w1414, offset (0)=0, length (rest)=2 ("length (rest)")) -> (substring=w1424:string)
          n649 = String Subset(string=w1414, offset (0)=3, length (rest)=2 ("length (rest)")) -> (substring=w1423:string)
          n650 = String Subset(string=w1414, offset (0)=6, length (rest)=2 ("length (rest)")) -> (substring=w1416:string)
          n651 = String Subset(string=w1414, offset (0)=9, length (rest)=2 ("length (rest)")) -> (substring=w1415:string)
          n652 = Index Array(array=w1410, index=66) -> (element=w1412:string)
          n653 = Concatenate Strings(w1424, w1423, w1416, w1415) -> (w1422:string)
          n654 = Hexadecimal String To Number(string=w1422) -> (number=w1421:u32)  [unwired: 2 in, 1 out]
          n655 = To Long Integer(number=w1421) -> (32bit integer=w1409:i32)
          n656 = Number To Decimal String(number=w1409) -> (decimal integer string=w1408:string)  [unwired: 1 in]
          n657 = Build Array(w1412, w1408) -> (w1411:string[])
          n658 = Build Array(w1411) -> (w1407:string[][])
        }
        frame 62218 {
          # "Shaft Speed (RPM) (0xF30A)"
          n659 = Index Array(array=w1431, index=67) -> (element=w1433:string)
          n660 = Build Array(w1433, w1429) -> (w1432:string[])
          n661 = Build Array(w1432) -> (w1430:string[][])
        }
        frame 62219 {
          # "Basket Speed (RPM) (0xF30B)"
          # "Check"
          n662 = Index Array(array=w1437, index=68) -> (element=w1439:string)
          n663 = Build Array(w1439, w1435) -> (w1438:string[])
          n664 = Build Array(w1438) -> (w1436:string[][])
        }
        frame 62221 {
          # "Current RMS (Amps) (0xF30D)"
          n665 = Fract/Exp String To Number(string=w1442) -> (number=w1441:dbl)  [unwired: 3 in, 1 out]
          n666 = Index Array(array=w1444, index=69) -> (element=w1448:string)
          n667 = Divide(x=w1441, y=1024.0) -> (x/y=w1446:dbl)
          n668 = Number To Fractional String(number=w1446) -> (F-format string=w1445:string)  [unwired: 3 in]
          n669 = Build Array(w1448, w1445) -> (w1447:string[])
          n670 = Build Array(w1447) -> (w1443:string[][])
        }
        frame 62222 {
          # "Target Speed (RPM) (0xF30E)"
          # "Check"
          n671 = String Subset(string=w1458, offset (0)=0, length (rest)=2 ("length (rest)")) -> (substring=w1464:string)
          n672 = String Subset(string=w1458, offset (0)=3, length (rest)=2 ("length (rest)")) -> (substring=w1463:string)
          n673 = Index Array(array=w1452, index=70) -> (element=w1456:string)
          n674 = Concatenate Strings(w1464, w1463) -> (w1462:string)
          n675 = Hexadecimal String To Number(string=w1462) -> (number=w1461:u32)  [unwired: 2 in, 1 out]
          n676 = To Word Integer(number=w1461) -> (16bit integer=w1460:i16)
          n677 = Absolute Value(x=w1460) -> (abs(x)=w1459:i16)
          n678 = To Unsigned Word Integer(number=w1459) -> (unsigned 16bit integer=w1454:u16)
          n679 = Number To Decimal String(number=w1454) -> (decimal integer string=w1453:string)  [unwired: 1 in]
          n680 = Build Array(w1456, w1453) -> (w1455:string[])
          n681 = Build Array(w1455) -> (w1451:string[][])
        }
        frame 62227 {
          # "Motor Mode (0xF313)"
          # "Check"
          n682 = Decimal String To Number(string=w1475) -> (number=w1476:i32)  [unwired: 2 in, 1 out]
          n683 = Index Array(array=w1471, index=71) -> (element=w1473:string)
          n684 = case shown="4" w1476 {
            tunnel: ["Closed Loop" "Closed Loop Angle" "Open Loop" "Open Loop Angle" "Coasting" "Braking" "Idle"] -> w1470
            frame 0, Default {
            }
            frame 1 {
            }
            frame 2 {
            }
            frame 3 {
            }
            frame 4 {
            }
            frame 5 {
            }
            frame 6 {
            }
          }
          n685 = Build Array(w1473, w1470) -> (w1472:string[])
          n686 = Build Array(w1472) -> (w1469:string[][])
        }
        frame 62229 {
          # "OOB Detected in Acceleration (0xF315)"
          # "Check"
          n687 = Index Array(array=w1486, index=72) -> (element=w1488:string)
          n688 = Build Array(w1488, w1484) -> (w1487:string[])
          n689 = Build Array(w1487) -> (w1485:string[][])
        }
        frame 62230 {
          # "OOB Detected in S-S (0xF316)"
          # "Check"
          n690 = Index Array(array=w1492, index=73) -> (element=w1494:string)
          n691 = Build Array(w1494, w1490) -> (w1493:string[])
          n692 = Build Array(w1493) -> (w1491:string[][])
        }
        frame 62231 {
          # "OOB ReDistribution Required (0xF317)"
          # "Check"
          n693 = Index Array(array=w1498, index=74) -> (element=w1500:string)
          n694 = Build Array(w1500, w1496) -> (w1499:string[])
          n695 = Build Array(w1499) -> (w1497:string[][])
        }
        frame 62233 {
          # "Motor Profile Status (0xF319)\nMotor Profile (0xF319)"
          # "Check"
          # "Check"
          n696 = String Subset(string=w1513, offset (0)=3, length (rest)=2 ("length (rest)")) -> (substring=w1518:string)
          n697 = String Subset(string=w1513, offset (0)=0, length (rest)=2 ("length (rest)")) -> (substring=w1515:string)
          n698 = Index Array(array=w1505, index #1=75 ("index"), index #2=76 ("index")) -> (element #1=w1510:string, element #2=w1509:string)
          n699 = case shown="\"0B\"" w1518 {
            tunnel: ["Unknown" ("Profile Status") "Started" ("Profile Status") "Stopped" ("Profile Status") "Paused" ("Profile Status") "Resumed" ("Profile Status") "Selected" ("Profile Status") "Completed" ("Profile Status")] -> w1504
            frame "00", Default {
            }
            frame "06" {
            }
            frame "07" {
            }
            frame "08" {
            }
            frame "09" {
            }
            frame "0A" {
            }
            frame "0B" {
            }
          }
          n700 = Hexadecimal String To Number(string=w1515) -> (number=w1514:u32)  [unwired: 2 in, 1 out]
          n701 = Build Array(w1510, w1509) -> (w1508:string[])
          n702 = Number To Decimal String(number=w1514) -> (decimal integer string=w1503:string)  [unwired: 1 in]
          n703 = Build Array(w1504, w1503) -> (w1507:string[])
          n704 = Build Array(w1508, w1507) -> (w1506:string[][])
          n705 = Transpose 2D Array(2D array=w1506) -> (transposed array=w1502:string[][])
        }
        frame 62237 {
          # "Mode Shift Status (0xF31D)"
          # "Check"
          n706 = Decimal String To Number(string=w1534) -> (number=w1535:i32)  [unwired: 2 in, 1 out]
          n707 = Index Array(array=w1530, index=77) -> (element=w1532:string)
          n708 = case shown="4" w1535 {
            tunnel: ["Unknown" ("Motor Profile") "Agitate State" ("Motor Profile") "Spin State" ("Motor Profile") "Trans to Spin" ("Motor Profile") "Trans to Agitate" ("Motor Profile")] -> w1529
            frame 0, Default {
            }
            frame 1 {
            }
            frame 2 {
            }
            frame 3 {
            }
            frame 4 {
            }
          }
          n709 = Build Array(w1532, w1529) -> (w1531:string[])
          n710 = Build Array(w1531) -> (w1528:string[][])
        }
        frame 62241 {
          # "ME Relay (0xF321)"
          # "Check"
          n711 = Index Array(array=w1543, index=78) -> (element=w1545:string)
          n712 = Build Array(w1545, w1541) -> (w1544:string[])
          n713 = Build Array(w1544) -> (w1542:string[][])
        }
        frame 62242 {
          # "Mode Shift FB (0xF322)"
          # "Check"
          n714 = Index Array(array=w1549, index=79) -> (element=w1551:string)
          n715 = Build Array(w1551, w1547) -> (w1550:string[])
          n716 = Build Array(w1550) -> (w1548:string[][])
        }
        frame 62243 {
          # "MS Motor (0xF323)"
          # "Check"
          n717 = Index Array(array=w1555, index=80) -> (element=w1557:string)
          n718 = Build Array(w1557, w1553) -> (w1556:string[])
          n719 = Build Array(w1556) -> (w1554:string[][])
        }
        frame 62250 {
          # "Check"
          n720 = call "Q5 Format.vi"("Data (U16 or U32)"=w1565) -> ("Q5 Format Data"=w1559:string)  [unwired: 10 in]
          n721 = Index Array(array=w1561, index=85) -> (element=w1563:string)
          n722 = Build Array(w1563, w1559) -> (w1562:string[])
          n723 = Build Array(w1562) -> (w1560:string[][])
        }
        frame 62253 {
          # "Partial Coast Time (0xF32D)"
          # "Check"
          n724 = Index Array(array=w1568, index=81) -> (element=w1570:string)
          n725 = Build Array(w1570, w1566) -> (w1569:string[])
          n726 = Build Array(w1569) -> (w1567:string[][])
        }
        frame 62254 {
          # "Ramp Line Voltage (0xF32E)"
          # "Check"
          n727 = Index Array(array=w1575, index=82) -> (element=w1577:string)
          n728 = call "Q5 Format.vi"("Data (U16 or U32)"=w1573) -> ("Q5 Format Data"=w1572:string)  [unwired: 10 in]
          n729 = Build Array(w1577, w1572) -> (w1576:string[])
          n730 = Build Array(w1576) -> (w1574:string[][])
        }
        frame 61440 {
          # "Personality (0xF000)"
          n731 = Index Array(array=w1581, index=83) -> (element=w1583:string)
          n732 = Build Array(w1583, w1579) -> (w1582:string[])
          n733 = Build Array(w1582) -> (w1580:string[][])
        }
        frame 61463 {
          # "Reset Source (0xF017)"
          # "Check"
          # "Line Number"
          # "File Name CRC"
          n734 = String Subset(string=w1595, offset (0)=0, length (rest)=5 ("length (rest)")) -> (substring=w1591:string)
          n735 = String Subset(string=w1595, offset (0)=6, length (rest)=2 ("length (rest)")) -> (substring=w1600:string)
          n736 = String Subset(string=w1595, offset (0)=9, length (rest)=2 ("length (rest)")) -> (substring=w1601:string)
          n737 = Concatenate Strings(w1600, w1601) -> (w1602:string)
          n738 = Hexadecimal String To Number(string=w1602) -> (number=w1593:u32)  [unwired: 2 in, 1 out]
          n739 = Number To Decimal String(number=w1593) -> (decimal integer string=w1592:string)  [unwired: 1 in]
          n740 = call <vilib>:"Space Constant.vi"() -> ("String"=w1594:string)
          n741 = Index Array(array=w1586, index=84) -> (element=w1589:string)
          n742 = Concatenate Strings(w1591, w1594, w1592) -> (w1587:string)
          n743 = Build Array(w1589, w1587) -> (w1588:string[])
          n744 = Build Array(w1588) -> (w1585:string[][])
        }
      }
    }
  }
  "Array" <- w6
  n745 = disable-structure shown="Disabled" {
    frame Disabled {
      # "2015 ERD Array"
      n746 = Index Array(array="ERD Cross Reference List", index (row)=1) -> (element=w1605:T1[])  [unwired: 1 in]
      n747 = case shown="\"2017 Washer\"" {
        selector: _ -> [_ _]
        tunnel: _ -> [w1609 w1617]
        tunnel: [w1609 w1613] -> w1608
        tunnel: "ERD Cross Reference List" -> [_ w1616]
        tunnel: w1605 -> [_ w1610]
        frame Default {
        }
        frame "2017 Washer" {
          # "2017 ERD Array"
          # "The 2017 washer outputs the same data as the 2015....the software group just changed ALL of the ERDs!!!! Again!! :("
          n748 = Index Array(array=w1616, index (row)=0) -> (element=w1618:T1[])  [unwired: 1 in]
          n749 = for {
            tunnel: w1618 -> [w1627] mode=indexing
            tunnel: w1617 -> [w1625]
            tunnel: [w1624] -> w1615
            tunnel: [w1623] -> w1612 mode=indexing
            i -> [w1624]
            stop <- w1623 stop-if-true
            # "Find the 2017 ERD Number Index"
            n750 = Unbundle By Name(w1627) -> ("ERD Number"=w1626:u16)
            n751 = Equal?(x=w1626, y=w1625) -> (x = y?=w1623:bool)
          }
          n752 = Index Array(array=w1610, index=w1615) -> (element=w1614:T1)
          n753 = Or Array Elements(Boolean array=w1612) -> (logical OR=w1611:bool)
          n754 = case shown="True" w1611 {
            tunnel: w1614 -> [_ w1622]
            tunnel: [u16 0 ("ERD Number") w1621] -> w1613
            frame False {
            }
            frame True {
              n755 = Unbundle By Name(w1622) -> ("ERD Number"=w1621:u16)
            }
          }
        }
      }
      "ERD Number 2" <- w1608
    }
    frame Enabled {
    }
  }
  "Error Out" <- "Error In"
